vi "beta-3.0.0.vi"() -> ()   [LabVIEW 2016]
uses:
  <vilib>/FPGAPlugInAG/cRIO-9063/niLvFpga_Open_cRIO-9063.vi
  <vilib>/rvi/interface/common/dynamic/niFpgaDynamicAddResources.vi
  <vilib>/Utility/error.llb/Error Cluster From Error Code.vi
  <vilib>/rvi/errors/niLvFpgaAdjustHostInterfaceError.vi
  <vilib>/FPGAPlugInAG/Dynamic/niLvFpga_Close_Dynamic.vi
  <vilib>/rvi/interface/nirviOpenFPGA/nirviOpenFPGA.xnode
  FPGA Bitfiles/multi-functionpr_FPGATarget_multi-function-f_bsn-gyeHrfY.lvbitx
  <vilib>/rvi/interface/nirviReadWriteControl/nirviReadWriteControl.xnode
  <vilib>/rvi/interface/nirviCloseFPGA/nirviCloseFPGA.xnode
  NiFpgaLv.dll
  <vilib>/rvi/interface/Simulation/niFpgaSimulationCallBeginRW.vi
panel:
  out "change indicator":T1
  in  "Output Configuration":T2={"Channel0"={"function"=enum."OFF", "switch high"=3.5, "switch low"=0.0, "scan begin"=0.0, "scan end"=0.0, "scan step"=0.0, "and gate high"=3.5, "and gate low"=0.0, "or gate high"=3.5, "or gate low"=0.0, "main input"=enum."DIO0", "sub input"=enum."DIO0"}, "Channel1"={"function"=enum."OFF", "switch high"=3.5, "switch low"=0.0, "scan begin"=0.0, "scan end"=0.0, "scan step"=0.0, "and gate high"=3.5, "and gate low"=0.0, "or gate high"=3.5, "or gate low"=0.0, "main input"=enum."DIO0", "sub input"=enum."DIO0"}, "Channel2"={"function"=enum."OFF", "switch high"=3.5, "switch low"=0.0, "scan begin"=0.0, "scan end"=0.0, "scan step"=0.0, "and gate high"=3.5, "and gate low"=0.0, "or gate high"=3.5, "or gate low"=0.0, "main input"=enum."DIO0", "sub input"=enum."DIO0"}, "Channel3"={"function"=enum."OFF", "switch high"=3.5, "switch low"=0.0, "scan begin"=0.0, "scan end"=0.0, "scan step"=0.0, "and gate high"=3.5, "and gate low"=0.0, "or gate high"=3.5, "or gate low"=0.0, "main input"=enum."DIO0", "sub input"=enum."DIO0"}, "Channel4"={"function"=enum."OFF", "switch high"=3.5, "switch low"=0.0, "scan begin"=0.0, "scan end"=0.0, "scan step"=0.0, "and gate high"=3.5, "and gate low"=0.0, "or gate high"=3.5, "or gate low"=0.0, "main input"=enum."DIO0", "sub input"=enum."DIO0"}, "Channel5"={"function"=enum."OFF", "switch high"=3.5, "switch low"=0.0, "scan begin"=0.0, "scan end"=0.0, "scan step"=0.0, "and gate high"=3.5, "and gate low"=0.0, "or gate high"=3.5, "or gate low"=0.0, "main input"=enum."DIO0", "sub input"=enum."DIO0"}, "Channel6"={"function"=enum."OFF", "switch high"=3.5, "switch low"=0.0, "scan begin"=0.0, "scan end"=0.0, "scan step"=0.0, "and gate high"=3.5, "and gate low"=0.0, "or gate high"=3.5, "or gate low"=0.0, "main input"=enum."DIO0", "sub input"=enum."DIO0"}, "Channel7"={"function"=enum."OFF", "switch high"=3.5, "switch low"=0.0, "scan begin"=0.0, "scan end"=0.0, "scan step"=0.0, "and gate high"=3.5, "and gate low"=0.0, "or gate high"=3.5, "or gate low"=0.0, "main input"=enum."DIO0", "sub input"=enum."DIO0"}, "Channel8"={"function"=enum."OFF", "switch high"=3.5, "switch low"=0.0, "scan begin"=0.0, "scan end"=0.0, "scan step"=0.0, "and gate high"=3.5, "and gate low"=0.0, "or gate high"=3.5, "or gate low"=0.0, "main input"=enum."DIO0", "sub input"=enum."DIO0"}, "Channel9"={"function"=enum."OFF", "switch high"=3.5, "switch low"=0.0, "scan begin"=0.0, "scan end"=0.0, "scan step"=0.0, "and gate high"=3.5, "and gate low"=0.0, "or gate high"=3.5, "or gate low"=0.0, "main input"=enum."DIO0", "sub input"=enum."DIO0"}, "Channel10"={"function"=enum."OFF", "switch high"=3.5, "switch low"=0.0, "scan begin"=0.0, "scan end"=0.0, "scan step"=0.0, "and gate high"=3.5, "and gate low"=0.0, "or gate high"=3.5, "or gate low"=0.0, "main input"=enum."DIO0", "sub input"=enum."DIO0"}, "Channel11"={"function"=enum."OFF", "switch high"=3.5, "switch low"=0.0, "scan begin"=0.0, "scan end"=0.0, "scan step"=0.0, "and gate high"=3.5, "and gate low"=0.0, "or gate high"=3.5, "or gate low"=0.0, "main input"=enum."DIO0", "sub input"=enum."DIO0"}, "Channel12"={"function"=enum."OFF", "switch high"=3.5, "switch low"=0.0, "scan begin"=0.0, "scan end"=0.0, "scan step"=0.0, "and gate high"=3.5, "and gate low"=0.0, "or gate high"=3.5, "or gate low"=0.0, "main input"=enum."DIO0", "sub input"=enum."DIO0"}, "Channel13"={"function"=enum."OFF", "switch high"=3.5, "switch low"=0.0, "scan begin"=0.0, "scan end"=0.0, "scan step"=0.0, "and gate high"=3.5, "and gate low"=0.0, "or gate high"=3.5, "or gate low"=0.0, "main input"=enum."DIO0", "sub input"=enum."DIO0"}, "Channel14"={"function"=enum."OFF", "switch high"=3.5, "switch low"=0.0, "scan begin"=0.0, "scan end"=0.0, "scan step"=0.0, "and gate high"=3.5, "and gate low"=0.0, "or gate high"=3.5, "or gate low"=0.0, "main input"=enum."DIO0", "sub input"=enum."DIO0"}, "Channel15"={"function"=enum."OFF", "switch high"=3.5, "switch low"=0.0, "scan begin"=0.0, "scan end"=0.0, "scan step"=0.0, "and gate high"=3.5, "and gate low"=0.0, "or gate high"=3.5, "or gate low"=0.0, "main input"=enum."DIO0", "sub input"=enum."DIO0"}} {"Channel15"."or gate low" format="%#_17g"; "Channel15"."or gate high" format="%#_17g"; "Channel15"."and gate low" format="%#_17g"; "Channel15"."and gate high" format="%#_17g"; "Channel15"."scan step" format="%#_17g"; "Channel15"."scan end" format="%#_17g"; "Channel15"."scan begin" format="%#_17g"; "Channel15"."switch low" format="%#_17g"; "Channel15"."switch high" format="%#_17g"; "Channel14"."or gate low" format="%#_17g"; "Channel14"."or gate high" format="%#_17g"; "Channel14"."and gate low" format="%#_17g"; "Channel14"."and gate high" format="%#_17g"; "Channel14"."scan step" format="%#_17g"; "Channel14"."scan end" format="%#_17g"; "Channel14"."scan begin" format="%#_17g"; "Channel14"."switch low" format="%#_17g"; "Channel14"."switch high" format="%#_17g"; "Channel13"."or gate low" format="%#_17g"; "Channel13"."or gate high" format="%#_17g"; "Channel13"."and gate low" format="%#_17g"; "Channel13"."and gate high" format="%#_17g"; "Channel13"."scan step" format="%#_17g"; "Channel13"."scan end" format="%#_17g"; "Channel13"."scan begin" format="%#_17g"; "Channel13"."switch low" format="%#_17g"; "Channel13"."switch high" format="%#_17g"; "Channel12"."or gate low" format="%#_17g"; "Channel12"."or gate high" format="%#_17g"; "Channel12"."and gate low" format="%#_17g"; "Channel12"."and gate high" format="%#_17g"; "Channel12"."scan step" format="%#_17g"; "Channel12"."scan end" format="%#_17g"; "Channel12"."scan begin" format="%#_17g"; "Channel12"."switch low" format="%#_17g"; "Channel12"."switch high" format="%#_17g"; "Channel11"."or gate low" format="%#_17g"; "Channel11"."or gate high" format="%#_17g"; "Channel11"."and gate low" format="%#_17g"; "Channel11"."and gate high" format="%#_17g"; "Channel11"."scan step" format="%#_17g"; "Channel11"."scan end" format="%#_17g"; "Channel11"."scan begin" format="%#_17g"; "Channel11"."switch low" format="%#_17g"; "Channel11"."switch high" format="%#_17g"; "Channel10"."or gate low" format="%#_17g"; "Channel10"."or gate high" format="%#_17g"; "Channel10"."and gate low" format="%#_17g"; "Channel10"."and gate high" format="%#_17g"; "Channel10"."scan step" format="%#_17g"; "Channel10"."scan end" format="%#_17g"; "Channel10"."scan begin" format="%#_17g"; "Channel10"."switch low" format="%#_17g"; "Channel10"."switch high" format="%#_17g"; "Channel9"."or gate low" format="%#_17g"; "Channel9"."or gate high" format="%#_17g"; "Channel9"."and gate low" format="%#_17g"; "Channel9"."and gate high" format="%#_17g"; "Channel9"."scan step" format="%#_17g"; "Channel9"."scan end" format="%#_17g"; "Channel9"."scan begin" format="%#_17g"; "Channel9"."switch low" format="%#_17g"; "Channel9"."switch high" format="%#_17g"; "Channel8"."or gate low" format="%#_17g"; "Channel8"."or gate high" format="%#_17g"; "Channel8"."and gate low" format="%#_17g"; "Channel8"."and gate high" format="%#_17g"; "Channel8"."scan step" format="%#_17g"; "Channel8"."scan end" format="%#_17g"; "Channel8"."scan begin" format="%#_17g"; "Channel8"."switch low" format="%#_17g"; "Channel8"."switch high" format="%#_17g"; "Channel7"."or gate low" format="%#_17g"; "Channel7"."or gate high" format="%#_17g"; "Channel7"."and gate low" format="%#_17g"; "Channel7"."and gate high" format="%#_17g"; "Channel7"."scan step" format="%#_17g"; "Channel7"."scan end" format="%#_17g"; "Channel7"."scan begin" format="%#_17g"; "Channel7"."switch low" format="%#_17g"; "Channel7"."switch high" format="%#_17g"; "Channel6"."or gate low" format="%#_17g"; "Channel6"."or gate high" format="%#_17g"; "Channel6"."and gate low" format="%#_17g"; "Channel6"."and gate high" format="%#_17g"; "Channel6"."scan step" format="%#_17g"; "Channel6"."scan end" format="%#_17g"; "Channel6"."scan begin" format="%#_17g"; "Channel6"."switch low" format="%#_17g"; "Channel6"."switch high" format="%#_17g"; "Channel5"."or gate low" format="%#_17g"; "Channel5"."or gate high" format="%#_17g"; "Channel5"."and gate low" format="%#_17g"; "Channel5"."and gate high" format="%#_17g"; "Channel5"."scan step" format="%#_17g"; "Channel5"."scan end" format="%#_17g"; "Channel5"."scan begin" format="%#_17g"; "Channel5"."switch low" format="%#_17g"; "Channel5"."switch high" format="%#_17g"; "Channel4"."or gate low" format="%#_17g"; "Channel4"."or gate high" format="%#_17g"; "Channel4"."and gate low" format="%#_17g"; "Channel4"."and gate high" format="%#_17g"; "Channel4"."scan step" format="%#_17g"; "Channel4"."scan end" format="%#_17g"; "Channel4"."scan begin" format="%#_17g"; "Channel4"."switch low" format="%#_17g"; "Channel4"."switch high" format="%#_17g"; "Channel3"."or gate low" format="%#_17g"; "Channel3"."or gate high" format="%#_17g"; "Channel3"."and gate low" format="%#_17g"; "Channel3"."and gate high" format="%#_17g"; "Channel3"."scan step" format="%#_17g"; "Channel3"."scan end" format="%#_17g"; "Channel3"."scan begin" format="%#_17g"; "Channel3"."switch low" format="%#_17g"; "Channel3"."switch high" format="%#_17g"; "Channel2"."or gate low" format="%#_17g"; "Channel2"."or gate high" format="%#_17g"; "Channel2"."and gate low" format="%#_17g"; "Channel2"."and gate high" format="%#_17g"; "Channel2"."scan step" format="%#_17g"; "Channel2"."scan end" format="%#_17g"; "Channel2"."scan begin" format="%#_17g"; "Channel2"."switch low" format="%#_17g"; "Channel2"."switch high" format="%#_17g"; "Channel1"."or gate low" format="%#_17g"; "Channel1"."or gate high" format="%#_17g"; "Channel1"."and gate low" format="%#_17g"; "Channel1"."and gate high" format="%#_17g"; "Channel1"."scan step" format="%#_17g"; "Channel1"."scan end" format="%#_17g"; "Channel1"."scan begin" format="%#_17g"; "Channel1"."switch low" format="%#_17g"; "Channel1"."switch high" format="%#_17g"; "Channel0"."or gate low" format="%#_17g"; "Channel0"."or gate high" format="%#_17g"; "Channel0"."and gate low" format="%#_17g"; "Channel0"."and gate high" format="%#_17g"; "Channel0"."scan step" format="%#_17g"; "Channel0"."scan end" format="%#_17g"; "Channel0"."scan begin" format="%#_17g"; "Channel0"."switch low" format="%#_17g"; "Channel0"."switch high" format="%#_17g"}
  in  "Configure":bool
  in  "Load":bool
  out "State":enum16{"Loading", "Running"}(ring)
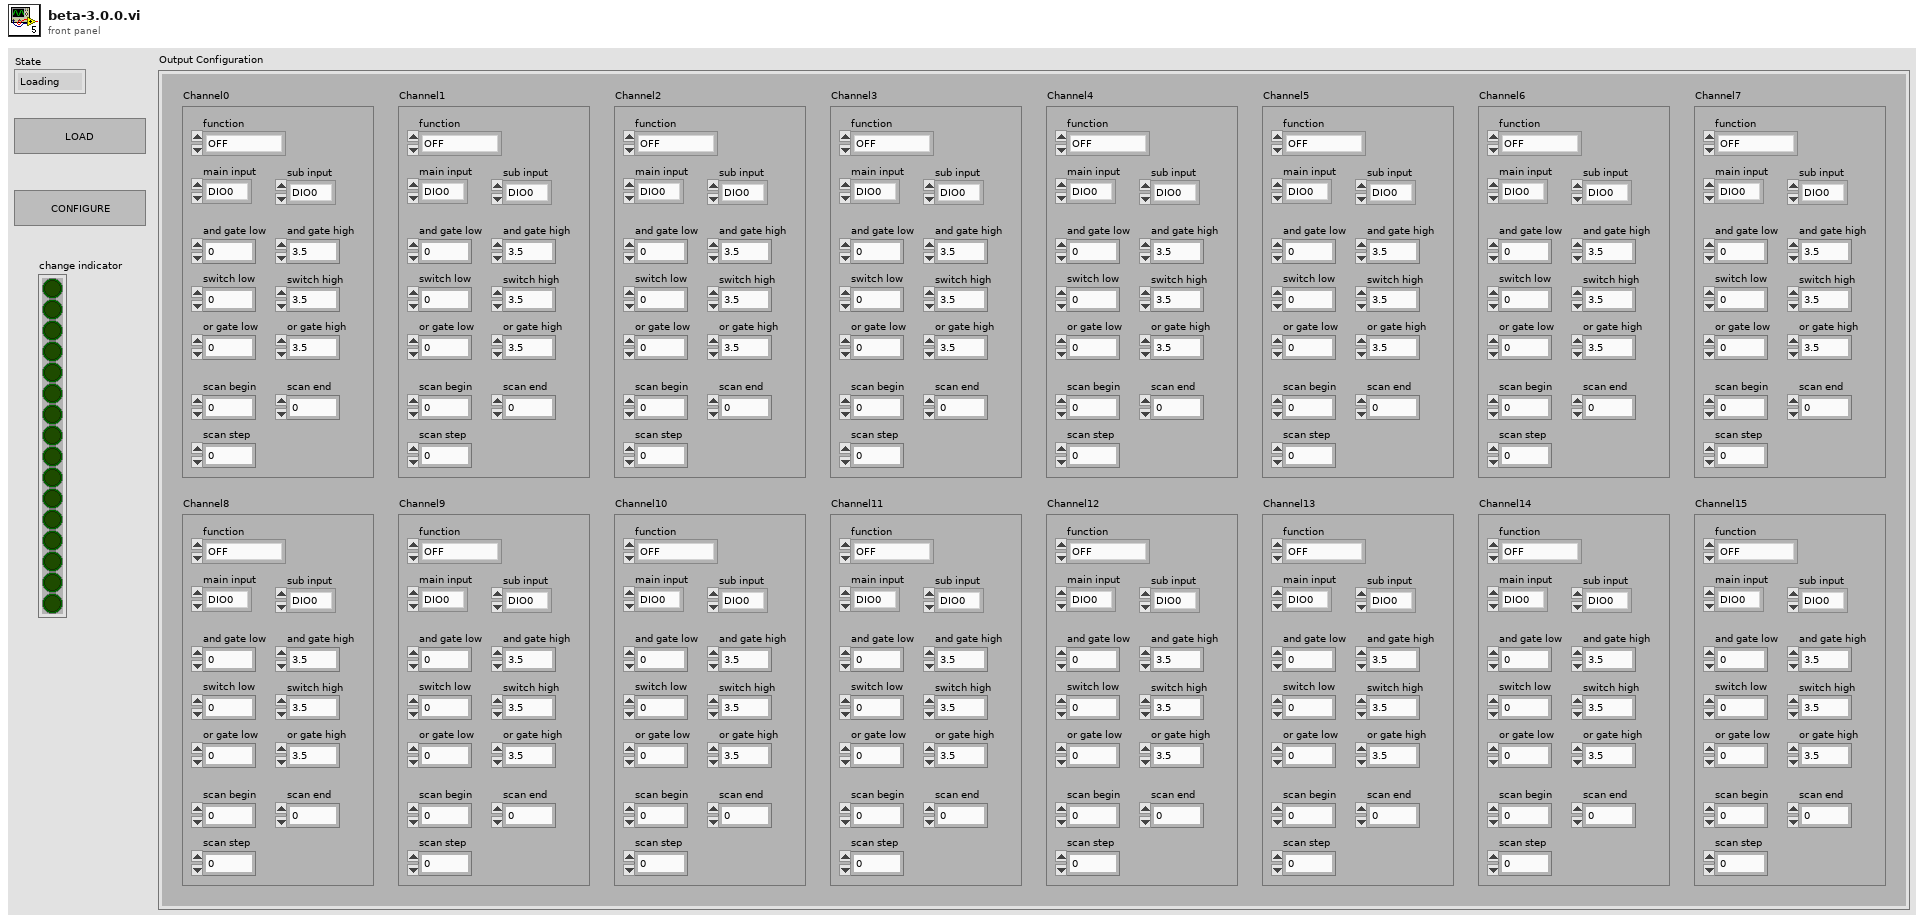
[diagram p1: front panel]
types:
  T1 = cluster{bool, bool, bool, bool, bool, bool, bool, bool, bool, bool, bool, bool, bool, bool, bool, bool}
  T2 = cluster{"Channel0":cluster{"function":enum16{"OFF", "SWITCH", "AND GATE", "OR GATE", "ITERATION"}, "switch high":sgl, "switch low":sgl, "scan begin":sgl, "scan end":sgl, "scan step":sgl, "and gate high":sgl, "and gate low":sgl, "or gate high":sgl, "or gate low":sgl, "main input":enum16{"DIO0", "DIO1", "DIO2", "DIO3", "DIO4", "DIO5", "DIO6", "DIO7", "DIO8", "DIO9", "DIO10", "DIO11", "DIO12", "DIO13", "DIO14", "DIO15", "DIO16", "DIO17", "DIO18", "DIO19", "DIO20", "DIO21", "DIO22", "DIO23", "DIO24", "DIO25", "DIO26", "DIO27", "DIO28", "DIO29", "DIO30", "DIO31"}, "sub input":enum16{"DIO0", "DIO1", "DIO2", "DIO3", "DIO4", "DIO5", "DIO6", "DIO7", "DIO8", "DIO9", "DIO10", "DIO11", "DIO12", "DIO13", "DIO14", "DIO15", "DIO16", "DIO17", "DIO18", "DIO19", "DIO20", "DIO21", "DIO22", "DIO23", "DIO24", "DIO25", "DIO26", "DIO27", "DIO28", "DIO29", "DIO30", "DIO31"}}, "Channel1":cluster{"function":enum16{"OFF", "SWITCH", "AND GATE", "OR GATE", "ITERATION"}, "switch high":sgl, "switch low":sgl, "scan begin":sgl, "scan end":sgl, "scan step":sgl, "and gate high":sgl, "and gate low":sgl, "or gate high":sgl, "or gate low":sgl, "main input":enum16{"DIO0", "DIO1", "DIO2", "DIO3", "DIO4", "DIO5", "DIO6", "DIO7", "DIO8", "DIO9", "DIO10", "DIO11", "DIO12", "DIO13", "DIO14", "DIO15", "DIO16", "DIO17", "DIO18", "DIO19", "DIO20", "DIO21", "DIO22", "DIO23", "DIO24", "DIO25", "DIO26", "DIO27", "DIO28", "DIO29", "DIO30", "DIO31"}, "sub input":enum16{"DIO0", "DIO1", "DIO2", "DIO3", "DIO4", "DIO5", "DIO6", "DIO7", "DIO8", "DIO9", "DIO10", "DIO11", "DIO12", "DIO13", "DIO14", "DIO15", "DIO16", "DIO17", "DIO18", "DIO19", "DIO20", "DIO21", "DIO22", "DIO23", "DIO24", "DIO25", "DIO26", "DIO27", "DIO28", "DIO29", "DIO30", "DIO31"}}, "Channel2":cluster{"function":enum16{"OFF", "SWITCH", "AND GATE", "OR GATE", "ITERATION"}, "switch high":sgl, "switch low":sgl, "scan begin":sgl, "scan end":sgl, "scan step":sgl, "and gate high":sgl, "and gate low":sgl, "or gate high":sgl, "or gate low":sgl, "main input":enum16{"DIO0", "DIO1", "DIO2", "DIO3", "DIO4", "DIO5", "DIO6", "DIO7", "DIO8", "DIO9", "DIO10", "DIO11", "DIO12", "DIO13", "DIO14", "DIO15", "DIO16", "DIO17", "DIO18", "DIO19", "DIO20", "DIO21", "DIO22", "DIO23", "DIO24", "DIO25", "DIO26", "DIO27", "DIO28", "DIO29", "DIO30", "DIO31"}, "sub input":enum16{"DIO0", "DIO1", "DIO2", "DIO3", "DIO4", "DIO5", "DIO6", "DIO7", "DIO8", "DIO9", "DIO10", "DIO11", "DIO12", "DIO13", "DIO14", "DIO15", "DIO16", "DIO17", "DIO18", "DIO19", "DIO20", "DIO21", "DIO22", "DIO23", "DIO24", "DIO25", "DIO26", "DIO27", "DIO28", "DIO29", "DIO30", "DIO31"}}, "Channel3":cluster{"function":enum16{"OFF", "SWITCH", "AND GATE", "OR GATE", "ITERATION"}, "switch high":sgl, "switch low":sgl, "scan begin":sgl, "scan end":sgl, "scan step":sgl, "and gate high":sgl, "and gate low":sgl, "or gate high":sgl, "or gate low":sgl, "main input":enum16{"DIO0", "DIO1", "DIO2", "DIO3", "DIO4", "DIO5", "DIO6", "DIO7", "DIO8", "DIO9", "DIO10", "DIO11", "DIO12", "DIO13", "DIO14", "DIO15", "DIO16", "DIO17", "DIO18", "DIO19", "DIO20", "DIO21", "DIO22", "DIO23", "DIO24", "DIO25", "DIO26", "DIO27", "DIO28", "DIO29", "DIO30", "DIO31"}, "sub input":enum16{"DIO0", "DIO1", "DIO2", "DIO3", "DIO4", "DIO5", "DIO6", "DIO7", "DIO8", "DIO9", "DIO10", "DIO11", "DIO12", "DIO13", "DIO14", "DIO15", "DIO16", "DIO17", "DIO18", "DIO19", "DIO20", "DIO21", "DIO22", "DIO23", "DIO24", "DIO25", "DIO26", "DIO27", "DIO28", "DIO29", "DIO30", "DIO31"}}, "Channel4":cluster{"function":enum16{"OFF", "SWITCH", "AND GATE", "OR GATE", "ITERATION"}, "switch high":sgl, "switch low":sgl, "scan begin":sgl, "scan end":sgl, "scan step":sgl, "and gate high":sgl, "and gate low":sgl, "or gate high":sgl, "or gate low":sgl, "main input":enum16{"DIO0", "DIO1", "DIO2", "DIO3", "DIO4", "DIO5", "DIO6", "DIO7", "DIO8", "DIO9", "DIO10", "DIO11", "DIO12", "DIO13", "DIO14", "DIO15", "DIO16", "DIO17", "DIO18", "DIO19", "DIO20", "DIO21", "DIO22", "DIO23", "DIO24", "DIO25", "DIO26", "DIO27", "DIO28", "DIO29", "DIO30", "DIO31"}, "sub input":enum16{"DIO0", "DIO1", "DIO2", "DIO3", "DIO4", "DIO5", "DIO6", "DIO7", "DIO8", "DIO9", "DIO10", "DIO11", "DIO12", "DIO13", "DIO14", "DIO15", "DIO16", "DIO17", "DIO18", "DIO19", "DIO20", "DIO21", "DIO22", "DIO23", "DIO24", "DIO25", "DIO26", "DIO27", "DIO28", "DIO29", "DIO30", "DIO31"}}, "Channel5":cluster{"function":enum16{"OFF", "SWITCH", "AND GATE", "OR GATE", "ITERATION"}, "switch high":sgl, "switch low":sgl, "scan begin":sgl, "scan end":sgl, "scan step":sgl, "and gate high":sgl, "and gate low":sgl, "or gate high":sgl, "or gate low":sgl, "main input":enum16{"DIO0", "DIO1", "DIO2", "DIO3", "DIO4", "DIO5", "DIO6", "DIO7", "DIO8", "DIO9", "DIO10", "DIO11", "DIO12", "DIO13", "DIO14", "DIO15", "DIO16", "DIO17", "DIO18", "DIO19", "DIO20", "DIO21", "DIO22", "DIO23", "DIO24", "DIO25", "DIO26", "DIO27", "DIO28", "DIO29", "DIO30", "DIO31"}, "sub input":enum16{"DIO0", "DIO1", "DIO2", "DIO3", "DIO4", "DIO5", "DIO6", "DIO7", "DIO8", "DIO9", "DIO10", "DIO11", "DIO12", "DIO13", "DIO14", "DIO15", "DIO16", "DIO17", "DIO18", "DIO19", "DIO20", "DIO21", "DIO22", "DIO23", "DIO24", "DIO25", "DIO26", "DIO27", "DIO28", "DIO29", "DIO30", "DIO31"}}, "Channel6":cluster{"function":enum16{"OFF", "SWITCH", "AND GATE", "OR GATE", "ITERATION"}, "switch high":sgl, "switch low":sgl, "scan begin":sgl, "scan end":sgl, "scan step":sgl, "and gate high":sgl, "and gate low":sgl, "or gate high":sgl, "or gate low":sgl, "main input":enum16{"DIO0", "DIO1", "DIO2", "DIO3", "DIO4", "DIO5", "DIO6", "DIO7", "DIO8", "DIO9", "DIO10", "DIO11", "DIO12", "DIO13", "DIO14", "DIO15", "DIO16", "DIO17", "DIO18", "DIO19", "DIO20", "DIO21", "DIO22", "DIO23", "DIO24", "DIO25", "DIO26", "DIO27", "DIO28", "DIO29", "DIO30", "DIO31"}, "sub input":enum16{"DIO0", "DIO1", "DIO2", "DIO3", "DIO4", "DIO5", "DIO6", "DIO7", "DIO8", "DIO9", "DIO10", "DIO11", "DIO12", "DIO13", "DIO14", "DIO15", "DIO16", "DIO17", "DIO18", "DIO19", "DIO20", "DIO21", "DIO22", "DIO23", "DIO24", "DIO25", "DIO26", "DIO27", "DIO28", "DIO29", "DIO30", "DIO31"}}, "Channel7":cluster{"function":enum16{"OFF", "SWITCH", "AND GATE", "OR GATE", "ITERATION"}, "switch high":sgl, "switch low":sgl, "scan begin":sgl, "scan end":sgl, "scan step":sgl, "and gate high":sgl, "and gate low":sgl, "or gate high":sgl, "or gate low":sgl, "main input":enum16{"DIO0", "DIO1", "DIO2", "DIO3", "DIO4", "DIO5", "DIO6", "DIO7", "DIO8", "DIO9", "DIO10", "DIO11", "DIO12", "DIO13", "DIO14", "DIO15", "DIO16", "DIO17", "DIO18", "DIO19", "DIO20", "DIO21", "DIO22", "DIO23", "DIO24", "DIO25", "DIO26", "DIO27", "DIO28", "DIO29", "DIO30", "DIO31"}, "sub input":enum16{"DIO0", "DIO1", "DIO2", "DIO3", "DIO4", "DIO5", "DIO6", "DIO7", "DIO8", "DIO9", "DIO10", "DIO11", "DIO12", "DIO13", "DIO14", "DIO15", "DIO16", "DIO17", "DIO18", "DIO19", "DIO20", "DIO21", "DIO22", "DIO23", "DIO24", "DIO25", "DIO26", "DIO27", "DIO28", "DIO29", "DIO30", "DIO31"}}, "Channel8":cluster{"function":enum16{"OFF", "SWITCH", "AND GATE", "OR GATE", "ITERATION"}, "switch high":sgl, "switch low":sgl, "scan begin":sgl, "scan end":sgl, "scan step":sgl, "and gate high":sgl, "and gate low":sgl, "or gate high":sgl, "or gate low":sgl, "main input":enum16{"DIO0", "DIO1", "DIO2", "DIO3", "DIO4", "DIO5", "DIO6", "DIO7", "DIO8", "DIO9", "DIO10", "DIO11", "DIO12", "DIO13", "DIO14", "DIO15", "DIO16", "DIO17", "DIO18", "DIO19", "DIO20", "DIO21", "DIO22", "DIO23", "DIO24", "DIO25", "DIO26", "DIO27", "DIO28", "DIO29", "DIO30", "DIO31"}, "sub input":enum16{"DIO0", "DIO1", "DIO2", "DIO3", "DIO4", "DIO5", "DIO6", "DIO7", "DIO8", "DIO9", "DIO10", "DIO11", "DIO12", "DIO13", "DIO14", "DIO15", "DIO16", "DIO17", "DIO18", "DIO19", "DIO20", "DIO21", "DIO22", "DIO23", "DIO24", "DIO25", "DIO26", "DIO27", "DIO28", "DIO29", "DIO30", "DIO31"}}, "Channel9":cluster{"function":enum16{"OFF", "SWITCH", "AND GATE", "OR GATE", "ITERATION"}, "switch high":sgl, "switch low":sgl, "scan begin":sgl, "scan end":sgl, "scan step":sgl, "and gate high":sgl, "and gate low":sgl, "or gate high":sgl, "or gate low":sgl, "main input":enum16{"DIO0", "DIO1", "DIO2", "DIO3", "DIO4", "DIO5", "DIO6", "DIO7", "DIO8", "DIO9", "DIO10", "DIO11", "DIO12", "DIO13", "DIO14", "DIO15", "DIO16", "DIO17", "DIO18", "DIO19", "DIO20", "DIO21", "DIO22", "DIO23", "DIO24", "DIO25", "DIO26", "DIO27", "DIO28", "DIO29", "DIO30", "DIO31"}, "sub input":enum16{"DIO0", "DIO1", "DIO2", "DIO3", "DIO4", "DIO5", "DIO6", "DIO7", "DIO8", "DIO9", "DIO10", "DIO11", "DIO12", "DIO13", "DIO14", "DIO15", "DIO16", "DIO17", "DIO18", "DIO19", "DIO20", "DIO21", "DIO22", "DIO23", "DIO24", "DIO25", "DIO26", "DIO27", "DIO28", "DIO29", "DIO30", "DIO31"}}, "Channel10":cluster{"function":enum16{"OFF", "SWITCH", "AND GATE", "OR GATE", "ITERATION"}, "switch high":sgl, "switch low":sgl, "scan begin":sgl, "scan end":sgl, "scan step":sgl, "and gate high":sgl, "and gate low":sgl, "or gate high":sgl, "or gate low":sgl, "main input":enum16{"DIO0", "DIO1", "DIO2", "DIO3", "DIO4", "DIO5", "DIO6", "DIO7", "DIO8", "DIO9", "DIO10", "DIO11", "DIO12", "DIO13", "DIO14", "DIO15", "DIO16", "DIO17", "DIO18", "DIO19", "DIO20", "DIO21", "DIO22", "DIO23", "DIO24", "DIO25", "DIO26", "DIO27", "DIO28", "DIO29", "DIO30", "DIO31"}, "sub input":enum16{"DIO0", "DIO1", "DIO2", "DIO3", "DIO4", "DIO5", "DIO6", "DIO7", "DIO8", "DIO9", "DIO10", "DIO11", "DIO12", "DIO13", "DIO14", "DIO15", "DIO16", "DIO17", "DIO18", "DIO19", "DIO20", "DIO21", "DIO22", "DIO23", "DIO24", "DIO25", "DIO26", "DIO27", "DIO28", "DIO29", "DIO30", "DIO31"}}, "Channel11":cluster{"function":enum16{"OFF", "SWITCH", "AND GATE", "OR GATE", "ITERATION"}, "switch high":sgl, "switch low":sgl, "scan begin":sgl, "scan end":sgl, "scan step":sgl, "and gate high":sgl, "and gate low":sgl, "or gate high":sgl, "or gate low":sgl, "main input":enum16{"DIO0", "DIO1", "DIO2", "DIO3", "DIO4", "DIO5", "DIO6", "DIO7", "DIO8", "DIO9", "DIO10", "DIO11", "DIO12", "DIO13", "DIO14", "DIO15", "DIO16", "DIO17", "DIO18", "DIO19", "DIO20", "DIO21", "DIO22", "DIO23", "DIO24", "DIO25", "DIO26", "DIO27", "DIO28", "DIO29", "DIO30", "DIO31"}, "sub input":enum16{"DIO0", "DIO1", "DIO2", "DIO3", "DIO4", "DIO5", "DIO6", "DIO7", "DIO8", "DIO9", "DIO10", "DIO11", "DIO12", "DIO13", "DIO14", "DIO15", "DIO16", "DIO17", "DIO18", "DIO19", "DIO20", "DIO21", "DIO22", "DIO23", "DIO24", "DIO25", "DIO26", "DIO27", "DIO28", "DIO29", "DIO30", "DIO31"}}, "Channel12":cluster{"function":enum16{"OFF", "SWITCH", "AND GATE", "OR GATE", "ITERATION"}, "switch high":sgl, "switch low":sgl, "scan begin":sgl, "scan end":sgl, "scan step":sgl, "and gate high":sgl, "and gate low":sgl, "or gate high":sgl, "or gate low":sgl, "main input":enum16{"DIO0", "DIO1", "DIO2", "DIO3", "DIO4", "DIO5", "DIO6", "DIO7", "DIO8", "DIO9", "DIO10", "DIO11", "DIO12", "DIO13", "DIO14", "DIO15", "DIO16", "DIO17", "DIO18", "DIO19", "DIO20", "DIO21", "DIO22", "DIO23", "DIO24", "DIO25", "DIO26", "DIO27", "DIO28", "DIO29", "DIO30", "DIO31"}, "sub input":enum16{"DIO0", "DIO1", "DIO2", "DIO3", "DIO4", "DIO5", "DIO6", "DIO7", "DIO8", "DIO9", "DIO10", "DIO11", "DIO12", "DIO13", "DIO14", "DIO15", "DIO16", "DIO17", "DIO18", "DIO19", "DIO20", "DIO21", "DIO22", "DIO23", "DIO24", "DIO25", "DIO26", "DIO27", "DIO28", "DIO29", "DIO30", "DIO31"}}, "Channel13":cluster{"function":enum16{"OFF", "SWITCH", "AND GATE", "OR GATE", "ITERATION"}, "switch high":sgl, "switch low":sgl, "scan begin":sgl, "scan end":sgl, "scan step":sgl, "and gate high":sgl, "and gate low":sgl, "or gate high":sgl, "or gate low":sgl, "main input":enum16{"DIO0", "DIO1", "DIO2", "DIO3", "DIO4", "DIO5", "DIO6", "DIO7", "DIO8", "DIO9", "DIO10", "DIO11", "DIO12", "DIO13", "DIO14", "DIO15", "DIO16", "DIO17", "DIO18", "DIO19", "DIO20", "DIO21", "DIO22", "DIO23", "DIO24", "DIO25", "DIO26", "DIO27", "DIO28", "DIO29", "DIO30", "DIO31"}, "sub input":enum16{"DIO0", "DIO1", "DIO2", "DIO3", "DIO4", "DIO5", "DIO6", "DIO7", "DIO8", "DIO9", "DIO10", "DIO11", "DIO12", "DIO13", "DIO14", "DIO15", "DIO16", "DIO17", "DIO18", "DIO19", "DIO20", "DIO21", "DIO22", "DIO23", "DIO24", "DIO25", "DIO26", "DIO27", "DIO28", "DIO29", "DIO30", "DIO31"}}, "Channel14":cluster{"function":enum16{"OFF", "SWITCH", "AND GATE", "OR GATE", "ITERATION"}, "switch high":sgl, "switch low":sgl, "scan begin":sgl, "scan end":sgl, "scan step":sgl, "and gate high":sgl, "and gate low":sgl, "or gate high":sgl, "or gate low":sgl, "main input":enum16{"DIO0", "DIO1", "DIO2", "DIO3", "DIO4", "DIO5", "DIO6", "DIO7", "DIO8", "DIO9", "DIO10", "DIO11", "DIO12", "DIO13", "DIO14", "DIO15", "DIO16", "DIO17", "DIO18", "DIO19", "DIO20", "DIO21", "DIO22", "DIO23", "DIO24", "DIO25", "DIO26", "DIO27", "DIO28", "DIO29", "DIO30", "DIO31"}, "sub input":enum16{"DIO0", "DIO1", "DIO2", "DIO3", "DIO4", "DIO5", "DIO6", "DIO7", "DIO8", "DIO9", "DIO10", "DIO11", "DIO12", "DIO13", "DIO14", "DIO15", "DIO16", "DIO17", "DIO18", "DIO19", "DIO20", "DIO21", "DIO22", "DIO23", "DIO24", "DIO25", "DIO26", "DIO27", "DIO28", "DIO29", "DIO30", "DIO31"}}, "Channel15":cluster{"function":enum16{"OFF", "SWITCH", "AND GATE", "OR GATE", "ITERATION"}, "switch high":sgl, "switch low":sgl, "scan begin":sgl, "scan end":sgl, "scan step":sgl, "and gate high":sgl, "and gate low":sgl, "or gate high":sgl, "or gate low":sgl, "main input":enum16{"DIO0", "DIO1", "DIO2", "DIO3", "DIO4", "DIO5", "DIO6", "DIO7", "DIO8", "DIO9", "DIO10", "DIO11", "DIO12", "DIO13", "DIO14", "DIO15", "DIO16", "DIO17", "DIO18", "DIO19", "DIO20", "DIO21", "DIO22", "DIO23", "DIO24", "DIO25", "DIO26", "DIO27", "DIO28", "DIO29", "DIO30", "DIO31"}, "sub input":enum16{"DIO0", "DIO1", "DIO2", "DIO3", "DIO4", "DIO5", "DIO6", "DIO7", "DIO8", "DIO9", "DIO10", "DIO11", "DIO12", "DIO13", "DIO14", "DIO15", "DIO16", "DIO17", "DIO18", "DIO19", "DIO20", "DIO21", "DIO22", "DIO23", "DIO24", "DIO25", "DIO26", "DIO27", "DIO28", "DIO29", "DIO30", "DIO31"}}}
  T3 = cluster{"Channel0":cluster{"function":bool, "switch high":bool, "switch low":bool, "scan begin":bool, "scan end":bool, "scan step":bool, "and gate high":bool, "and gate low":bool, "or gate high":bool, "or gate low":bool, "main input":bool, "sub input":bool}, "Channel1":cluster{"function":bool, "switch high":bool, "switch low":bool, "scan begin":bool, "scan end":bool, "scan step":bool, "and gate high":bool, "and gate low":bool, "or gate high":bool, "or gate low":bool, "main input":bool, "sub input":bool}, "Channel2":cluster{"function":bool, "switch high":bool, "switch low":bool, "scan begin":bool, "scan end":bool, "scan step":bool, "and gate high":bool, "and gate low":bool, "or gate high":bool, "or gate low":bool, "main input":bool, "sub input":bool}, "Channel3":cluster{"function":bool, "switch high":bool, "switch low":bool, "scan begin":bool, "scan end":bool, "scan step":bool, "and gate high":bool, "and gate low":bool, "or gate high":bool, "or gate low":bool, "main input":bool, "sub input":bool}, "Channel4":cluster{"function":bool, "switch high":bool, "switch low":bool, "scan begin":bool, "scan end":bool, "scan step":bool, "and gate high":bool, "and gate low":bool, "or gate high":bool, "or gate low":bool, "main input":bool, "sub input":bool}, "Channel5":cluster{"function":bool, "switch high":bool, "switch low":bool, "scan begin":bool, "scan end":bool, "scan step":bool, "and gate high":bool, "and gate low":bool, "or gate high":bool, "or gate low":bool, "main input":bool, "sub input":bool}, "Channel6":cluster{"function":bool, "switch high":bool, "switch low":bool, "scan begin":bool, "scan end":bool, "scan step":bool, "and gate high":bool, "and gate low":bool, "or gate high":bool, "or gate low":bool, "main input":bool, "sub input":bool}, "Channel7":cluster{"function":bool, "switch high":bool, "switch low":bool, "scan begin":bool, "scan end":bool, "scan step":bool, "and gate high":bool, "and gate low":bool, "or gate high":bool, "or gate low":bool, "main input":bool, "sub input":bool}, "Channel8":cluster{"function":bool, "switch high":bool, "switch low":bool, "scan begin":bool, "scan end":bool, "scan step":bool, "and gate high":bool, "and gate low":bool, "or gate high":bool, "or gate low":bool, "main input":bool, "sub input":bool}, "Channel9":cluster{"function":bool, "switch high":bool, "switch low":bool, "scan begin":bool, "scan end":bool, "scan step":bool, "and gate high":bool, "and gate low":bool, "or gate high":bool, "or gate low":bool, "main input":bool, "sub input":bool}, "Channel10":cluster{"function":bool, "switch high":bool, "switch low":bool, "scan begin":bool, "scan end":bool, "scan step":bool, "and gate high":bool, "and gate low":bool, "or gate high":bool, "or gate low":bool, "main input":bool, "sub input":bool}, "Channel11":cluster{"function":bool, "switch high":bool, "switch low":bool, "scan begin":bool, "scan end":bool, "scan step":bool, "and gate high":bool, "and gate low":bool, "or gate high":bool, "or gate low":bool, "main input":bool, "sub input":bool}, "Channel12":cluster{"function":bool, "switch high":bool, "switch low":bool, "scan begin":bool, "scan end":bool, "scan step":bool, "and gate high":bool, "and gate low":bool, "or gate high":bool, "or gate low":bool, "main input":bool, "sub input":bool}, "Channel13":cluster{"function":bool, "switch high":bool, "switch low":bool, "scan begin":bool, "scan end":bool, "scan step":bool, "and gate high":bool, "and gate low":bool, "or gate high":bool, "or gate low":bool, "main input":bool, "sub input":bool}, "Channel14":cluster{"function":bool, "switch high":bool, "switch low":bool, "scan begin":bool, "scan end":bool, "scan step":bool, "and gate high":bool, "and gate low":bool, "or gate high":bool, "or gate low":bool, "main input":bool, "sub input":bool}, "Channel15":cluster{"function":bool, "switch high":bool, "switch low":bool, "scan begin":bool, "scan end":bool, "scan step":bool, "and gate high":bool, "and gate low":bool, "or gate high":bool, "or gate low":bool, "main input":bool, "sub input":bool}}
  T4 = cluster{"function":bool, "switch high":bool, "switch low":bool, "scan begin":bool, "scan end":bool, "scan step":bool, "and gate high":bool, "and gate low":bool, "or gate high":bool, "or gate low":bool, "main input":bool, "sub input":bool}
  T5 = cluster{"function":enum16{"OFF", "SWITCH", "AND GATE", "OR GATE", "ITERATION"}, "switch high":sgl, "switch low":sgl, "scan begin":sgl, "scan end":sgl, "scan step":sgl, "and gate high":sgl, "and gate low":sgl, "or gate high":sgl, "or gate low":sgl, "main input":enum16{"DIO0", "DIO1", "DIO2", "DIO3", "DIO4", "DIO5", "DIO6", "DIO7", "DIO8", "DIO9", "DIO10", "DIO11", "DIO12", "DIO13", "DIO14", "DIO15", "DIO16", "DIO17", "DIO18", "DIO19", "DIO20", "DIO21", "DIO22", "DIO23", "DIO24", "DIO25", "DIO26", "DIO27", "DIO28", "DIO29", "DIO30", "DIO31"}, "sub input":enum16{"DIO0", "DIO1", "DIO2", "DIO3", "DIO4", "DIO5", "DIO6", "DIO7", "DIO8", "DIO9", "DIO10", "DIO11", "DIO12", "DIO13", "DIO14", "DIO15", "DIO16", "DIO17", "DIO18", "DIO19", "DIO20", "DIO21", "DIO22", "DIO23", "DIO24", "DIO25", "DIO26", "DIO27", "DIO28", "DIO29", "DIO30", "DIO31"}}
  T6 = enum16{"OFF", "SWITCH", "AND GATE", "OR GATE", "ITERATION"}
  T7 = enum16{"DIO0", "DIO1", "DIO2", "DIO3", "DIO4", "DIO5", "DIO6", "DIO7", "DIO8", "DIO9", "DIO10", "DIO11", "DIO12", "DIO13", "DIO14", "DIO15", "DIO16", "DIO17", "DIO18", "DIO19", "DIO20", "DIO21", "DIO22", "DIO23", "DIO24", "DIO25", "DIO26", "DIO27", "DIO28", "DIO29", "DIO30", "DIO31"}
  T8 = cluster{"function":enum16{"OFF", "SWITCH", "AND GATE", "OR GATE", "ITERATION"}, "scan end":sgl, "scan begin":sgl, "scan step":sgl, bool, "main input":enum16{"DIO0", "DIO1", "DIO2", "DIO3", "DIO4", "DIO5", "DIO6", "DIO7", "DIO8", "DIO9", "DIO10", "DIO11", "DIO12", "DIO13", "DIO14", "DIO15", "DIO16", "DIO17", "DIO18", "DIO19", "DIO20", "DIO21", "DIO22", "DIO23", "DIO24", "DIO25", "DIO26", "DIO27", "DIO28", "DIO29", "DIO30", "DIO31"}, "sub input":enum16{"DIO0", "DIO1", "DIO2", "DIO3", "DIO4", "DIO5", "DIO6", "DIO7", "DIO8", "DIO9", "DIO10", "DIO11", "DIO12", "DIO13", "DIO14", "DIO15", "DIO16", "DIO17", "DIO18", "DIO19", "DIO20", "DIO21", "DIO22", "DIO23", "DIO24", "DIO25", "DIO26", "DIO27", "DIO28", "DIO29", "DIO30", "DIO31"}}
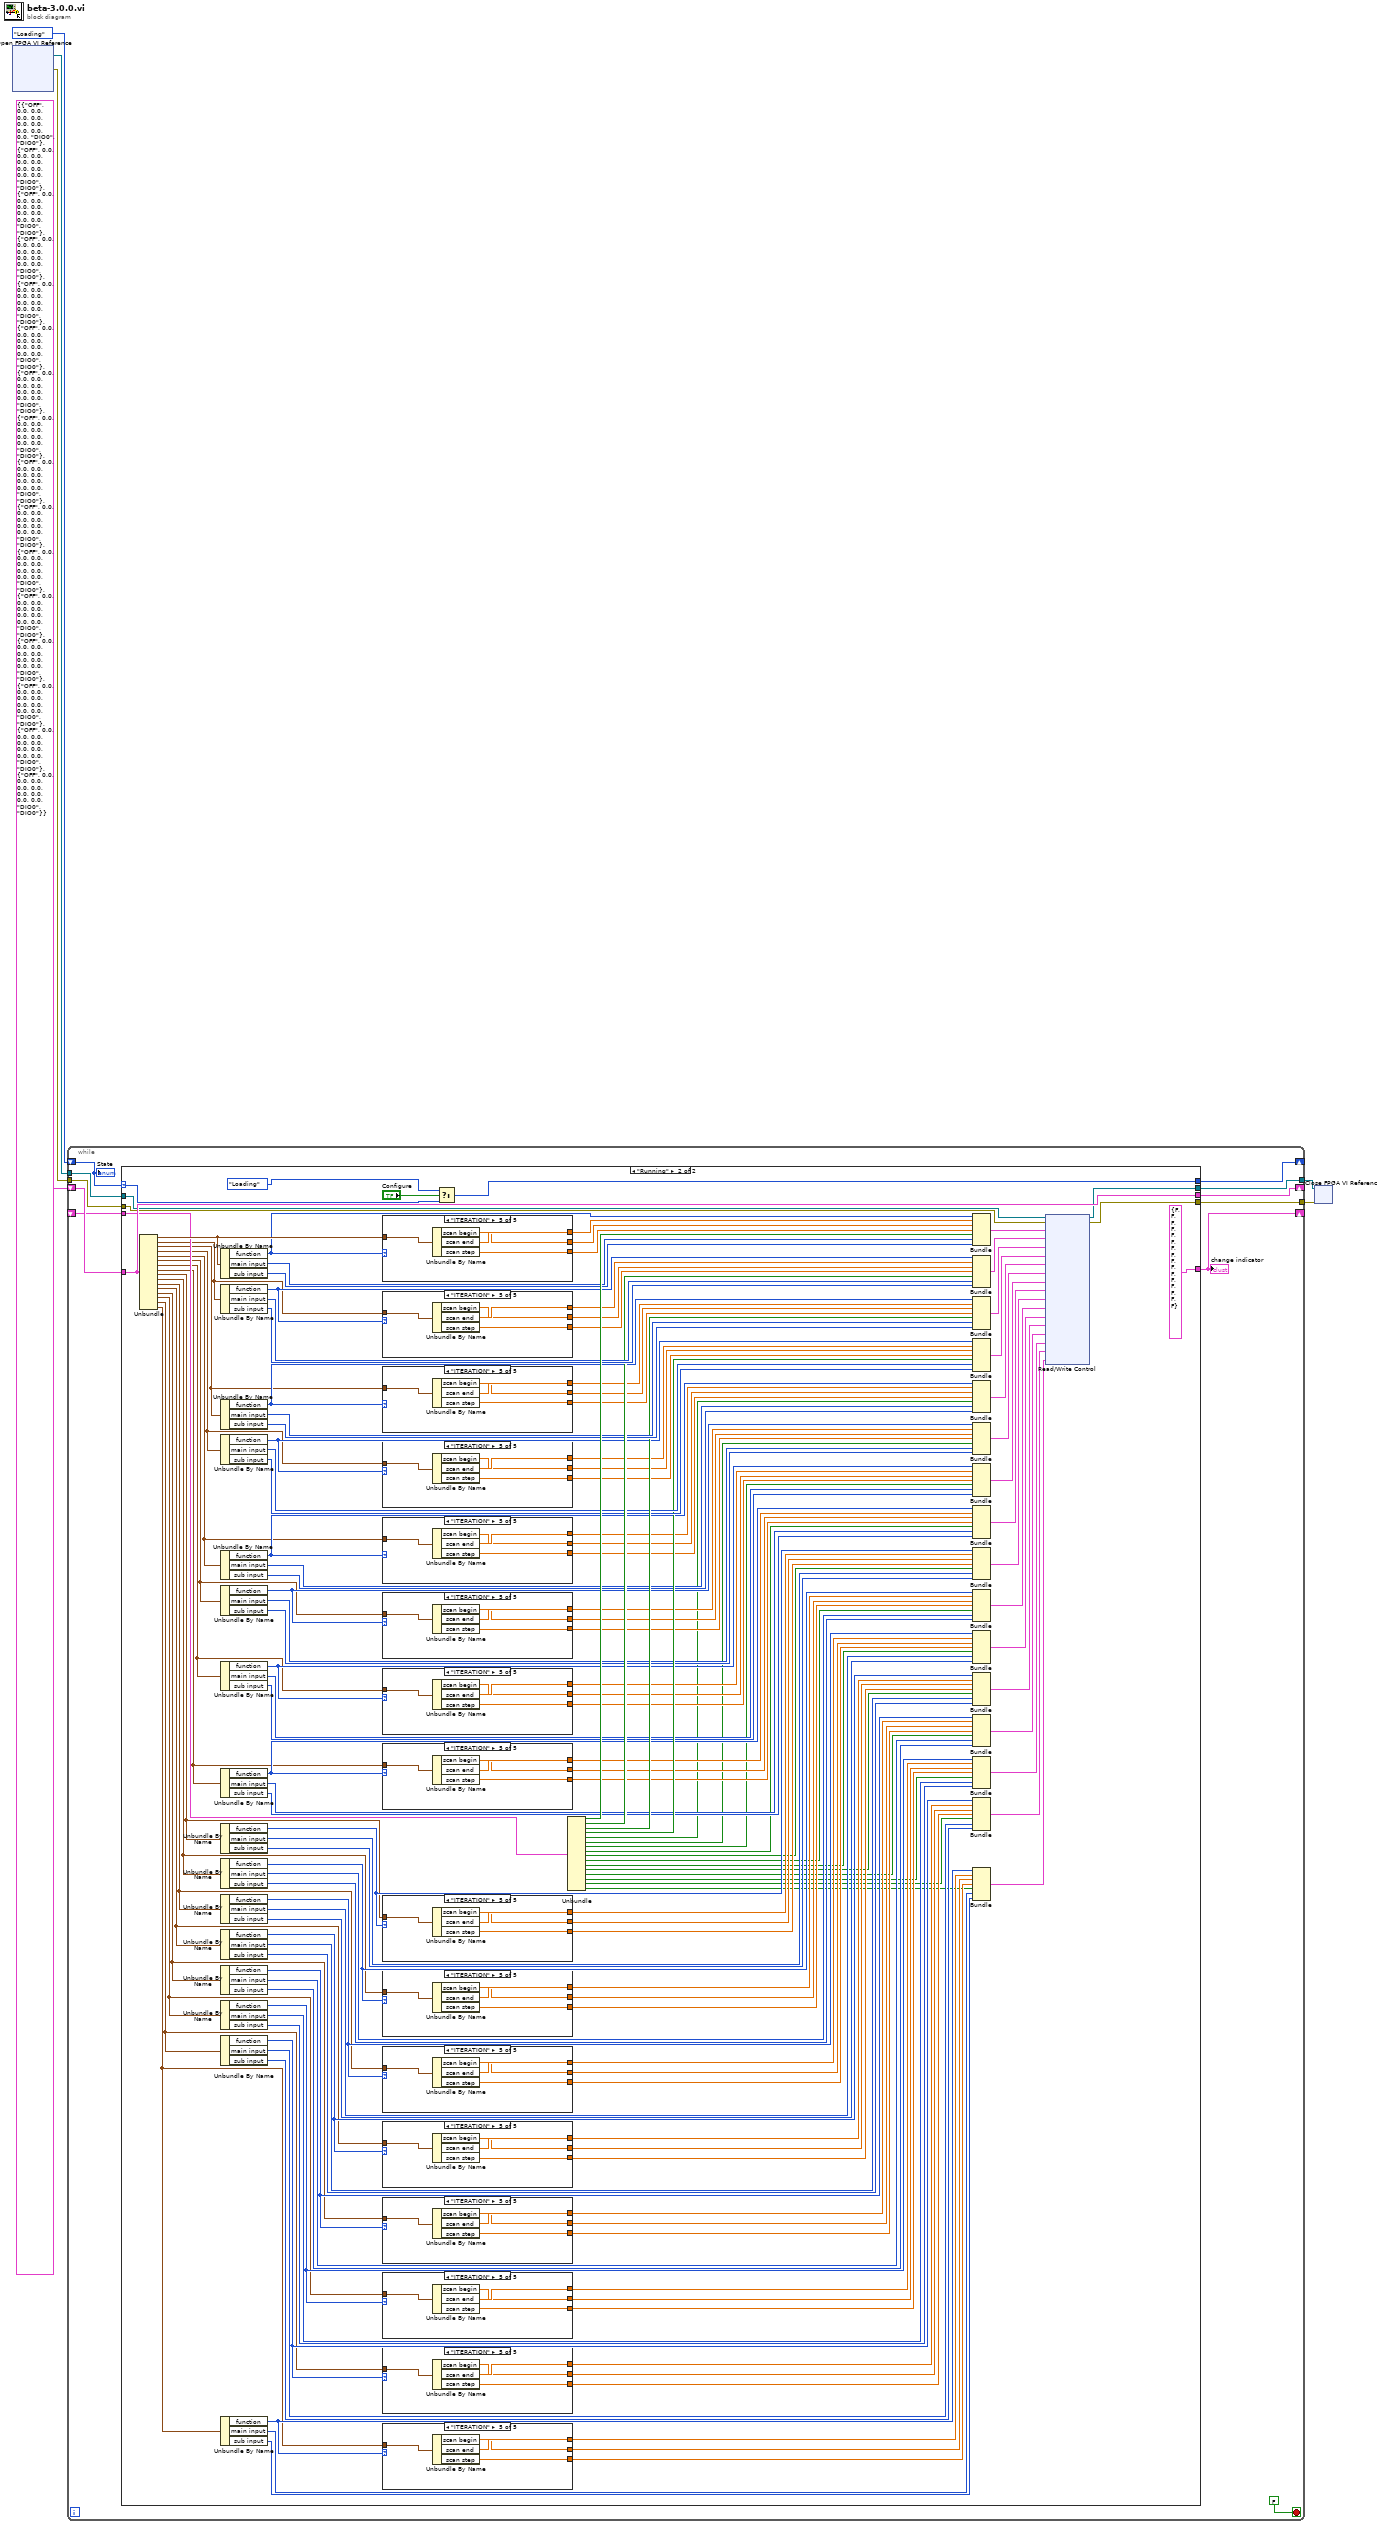
[diagram p0: block diagram]
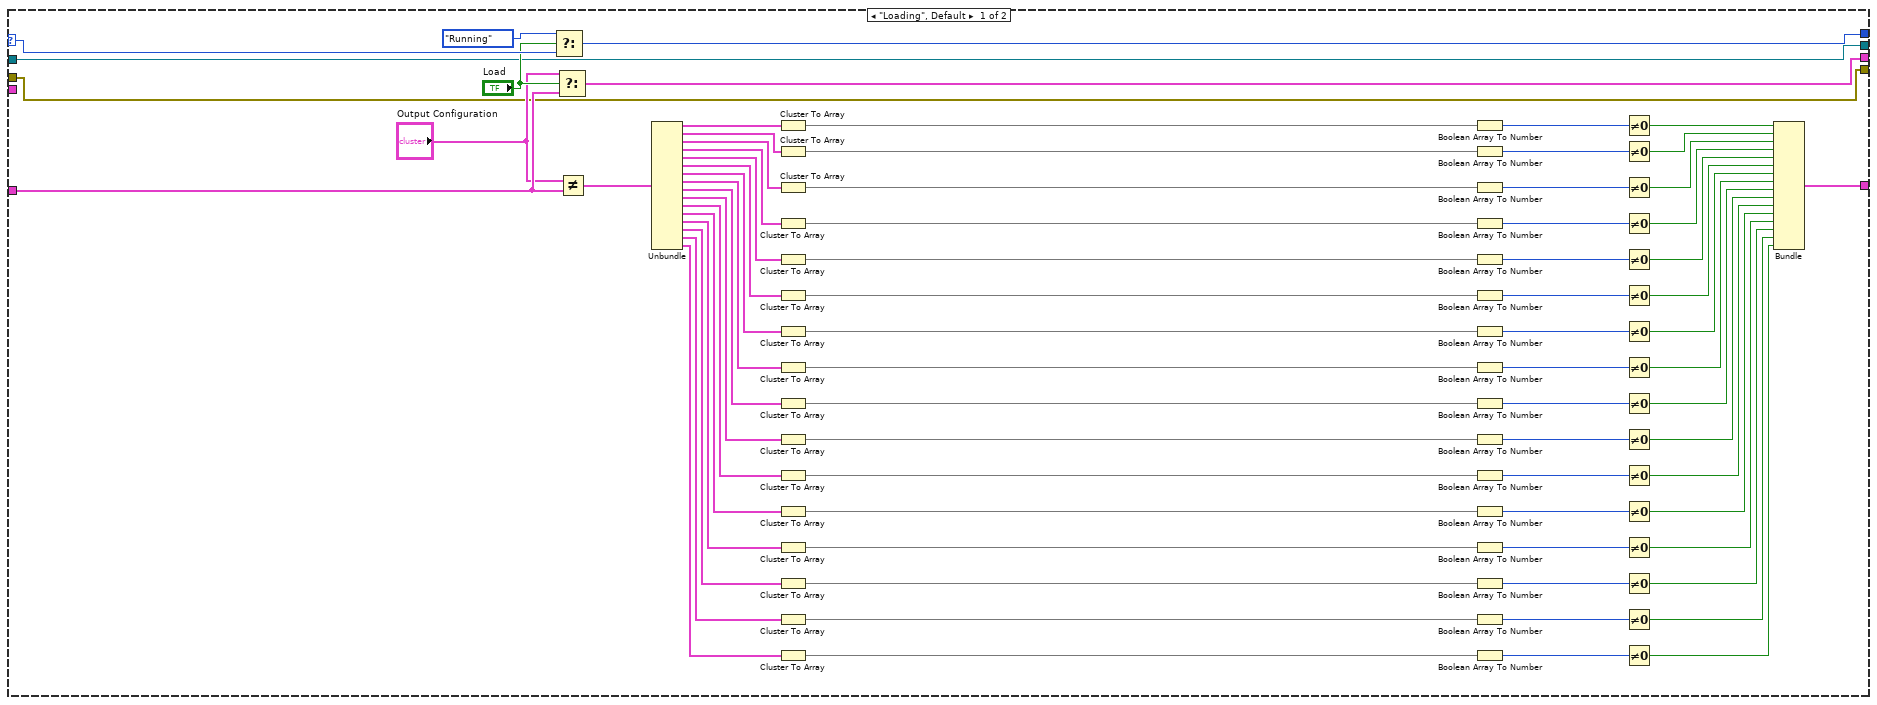
[diagram p2: hidden frame]
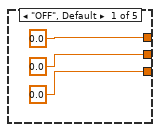
[diagram p3: hidden frame]
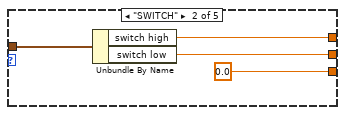
[diagram p4: hidden frame]
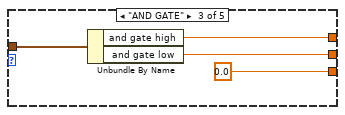
[diagram p5: hidden frame]
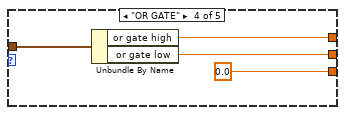
[diagram p6: hidden frame]
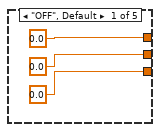
[diagram p7: hidden frame]
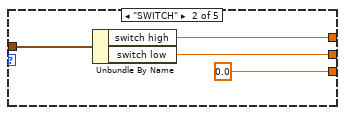
[diagram p8: hidden frame]
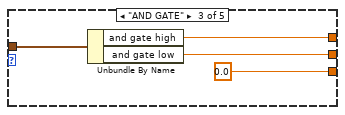
[diagram p9: hidden frame]
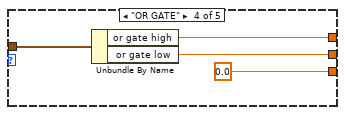
[diagram p10: hidden frame]
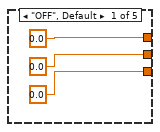
[diagram p11: hidden frame]
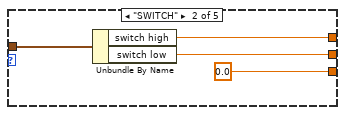
[diagram p12: hidden frame]
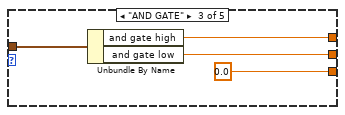
[diagram p13: hidden frame]
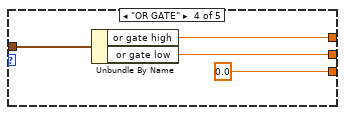
[diagram p14: hidden frame]
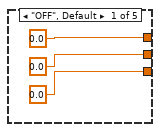
[diagram p15: hidden frame]
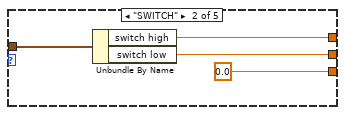
[diagram p16: hidden frame]
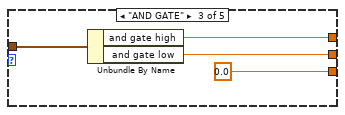
[diagram p17: hidden frame]
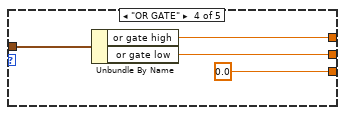
[diagram p18: hidden frame]
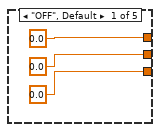
[diagram p19: hidden frame]
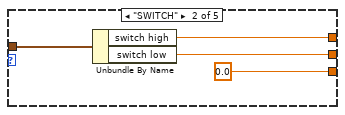
[diagram p20: hidden frame]
diagram:
  n1 = xnode "Open FPGA VI Reference"() -> ("FPGA VI Reference Out"=w4:refnum<k20>, "error out"=w3:errorcluster)  [unwired: 2 in]
  n2 = while {
    shift-right: [w14] -> _
    shift-left: T2 {"Channel0"={"function"=enum."OFF", "switch high"=0.0, "switch low"=0.0, "scan begin"=0.0, "scan end"=0.0, "scan step"=0.0, "and gate high"=0.0, "and gate low"=0.0, "or gate high"=0.0, "or gate low"=0.0, "main input"=enum."DIO0", "sub input"=enum."DIO0"}, "Channel1"={"function"=enum."OFF", "switch high"=0.0, "switch low"=0.0, "scan begin"=0.0, "scan end"=0.0, "scan step"=0.0, "and gate high"=0.0, "and gate low"=0.0, "or gate high"=0.0, "or gate low"=0.0, "main input"=enum."DIO0", "sub input"=enum."DIO0"}, "Channel2"={"function"=enum."OFF", "switch high"=0.0, "switch low"=0.0, "scan begin"=0.0, "scan end"=0.0, "scan step"=0.0, "and gate high"=0.0, "and gate low"=0.0, "or gate high"=0.0, "or gate low"=0.0, "main input"=enum."DIO0", "sub input"=enum."DIO0"}, "Channel3"={"function"=enum."OFF", "switch high"=0.0, "switch low"=0.0, "scan begin"=0.0, "scan end"=0.0, "scan step"=0.0, "and gate high"=0.0, "and gate low"=0.0, "or gate high"=0.0, "or gate low"=0.0, "main input"=enum."DIO0", "sub input"=enum."DIO0"}, "Channel4"={"function"=enum."OFF", "switch high"=0.0, "switch low"=0.0, "scan begin"=0.0, "scan end"=0.0, "scan step"=0.0, "and gate high"=0.0, "and gate low"=0.0, "or gate high"=0.0, "or gate low"=0.0, "main input"=enum."DIO0", "sub input"=enum."DIO0"}, "Channel5"={"function"=enum."OFF", "switch high"=0.0, "switch low"=0.0, "scan begin"=0.0, "scan end"=0.0, "scan step"=0.0, "and gate high"=0.0, "and gate low"=0.0, "or gate high"=0.0, "or gate low"=0.0, "main input"=enum."DIO0", "sub input"=enum."DIO0"}, "Channel6"={"function"=enum."OFF", "switch high"=0.0, "switch low"=0.0, "scan begin"=0.0, "scan end"=0.0, "scan step"=0.0, "and gate high"=0.0, "and gate low"=0.0, "or gate high"=0.0, "or gate low"=0.0, "main input"=enum."DIO0", "sub input"=enum."DIO0"}, "Channel7"={"function"=enum."OFF", "switch high"=0.0, "switch low"=0.0, "scan begin"=0.0, "scan end"=0.0, "scan step"=0.0, "and gate high"=0.0, "and gate low"=0.0, "or gate high"=0.0, "or gate low"=0.0, "main input"=enum."DIO0", "sub input"=enum."DIO0"}, "Channel8"={"function"=enum."OFF", "switch high"=0.0, "switch low"=0.0, "scan begin"=0.0, "scan end"=0.0, "scan step"=0.0, "and gate high"=0.0, "and gate low"=0.0, "or gate high"=0.0, "or gate low"=0.0, "main input"=enum."DIO0", "sub input"=enum."DIO0"}, "Channel9"={"function"=enum."OFF", "switch high"=0.0, "switch low"=0.0, "scan begin"=0.0, "scan end"=0.0, "scan step"=0.0, "and gate high"=0.0, "and gate low"=0.0, "or gate high"=0.0, "or gate low"=0.0, "main input"=enum."DIO0", "sub input"=enum."DIO0"}, "Channel10"={"function"=enum."OFF", "switch high"=0.0, "switch low"=0.0, "scan begin"=0.0, "scan end"=0.0, "scan step"=0.0, "and gate high"=0.0, "and gate low"=0.0, "or gate high"=0.0, "or gate low"=0.0, "main input"=enum."DIO0", "sub input"=enum."DIO0"}, "Channel11"={"function"=enum."OFF", "switch high"=0.0, "switch low"=0.0, "scan begin"=0.0, "scan end"=0.0, "scan step"=0.0, "and gate high"=0.0, "and gate low"=0.0, "or gate high"=0.0, "or gate low"=0.0, "main input"=enum."DIO0", "sub input"=enum."DIO0"}, "Channel12"={"function"=enum."OFF", "switch high"=0.0, "switch low"=0.0, "scan begin"=0.0, "scan end"=0.0, "scan step"=0.0, "and gate high"=0.0, "and gate low"=0.0, "or gate high"=0.0, "or gate low"=0.0, "main input"=enum."DIO0", "sub input"=enum."DIO0"}, "Channel13"={"function"=enum."OFF", "switch high"=0.0, "switch low"=0.0, "scan begin"=0.0, "scan end"=0.0, "scan step"=0.0, "and gate high"=0.0, "and gate low"=0.0, "or gate high"=0.0, "or gate low"=0.0, "main input"=enum."DIO0", "sub input"=enum."DIO0"}, "Channel14"={"function"=enum."OFF", "switch high"=0.0, "switch low"=0.0, "scan begin"=0.0, "scan end"=0.0, "scan step"=0.0, "and gate high"=0.0, "and gate low"=0.0, "or gate high"=0.0, "or gate low"=0.0, "main input"=enum."DIO0", "sub input"=enum."DIO0"}, "Channel15"={"function"=enum."OFF", "switch high"=0.0, "switch low"=0.0, "scan begin"=0.0, "scan end"=0.0, "scan step"=0.0, "and gate high"=0.0, "and gate low"=0.0, "or gate high"=0.0, "or gate low"=0.0, "main input"=enum."DIO0", "sub input"=enum."DIO0"}} ("Output Configuration") -> [w13]
    shift-right: [w16] -> _
    shift-left: enum16{"Loading", "Running"}."Loading" ("State") -> [w15]
    shift-right: [w12] -> _
    shift-left: _ -> [w7]
    tunnel: w4 -> [w11]
    tunnel: w3 -> [w10]
    tunnel: [w9] -> w2
    tunnel: [w8] -> w1
    stop <- FALSE stop-if-true
    n3 = case shown="\"Running\"" w15 {
      selector: w15 -> [w92 w244]
      tunnel: [w91 w246] -> w16
      tunnel: [w85 w242] -> w14
      tunnel: w13 -> [w87 w242]
      tunnel: [w20 T1 {FALSE, FALSE, FALSE, FALSE, FALSE, FALSE, FALSE, FALSE, FALSE, FALSE, FALSE, FALSE, FALSE, FALSE, FALSE, FALSE}] -> w12
      tunnel: w11 -> [w19 w240]
      tunnel: w10 -> [w18 w239]
      tunnel: [w19 w238] -> w9
      tunnel: [w18 w237] -> w8
      tunnel: w7 -> [_ w232]
      frame "Loading", Default {
        n4 = Select(t=enum16{"Loading", "Running"}."Running", s="Load", f=w92) -> (s? t:f=w91:enum16{"Loading", "Running"})
        n5 = Select(t="Output Configuration", s="Load", f=w87) -> (s? t:f=w85:T2)
        n6 = Not Equal?(x="Output Configuration", y=w87) -> (x != y?=w89:T3)
        n7 = Unbundle(w89) -> ("Channel0"=w52:T4, "Channel1"=w51:T4, "Channel2"=w50:T4, "Channel3"=w49:T4, "Channel4"=w48:T4, "Channel5"=w47:T4, "Channel6"=w46:T4, "Channel7"=w45:T4, "Channel8"=w44:T4, "Channel9"=w43:T4, "Channel10"=w42:T4, "Channel11"=w41:T4, "Channel12"=w40:T4, "Channel13"=w39:T4, "Channel14"=w38:T4, "Channel15"=w37:T4)
        n8 = Cluster To Array(cluster=w52) -> (array=w62:bool[])
        n9 = Cluster To Array(cluster=w51) -> (array=w64:bool[])
        n10 = Cluster To Array(cluster=w50) -> (array=w66:bool[])
        n11 = Cluster To Array(cluster=w49) -> (array=w68:bool[])
        n12 = Cluster To Array(cluster=w48) -> (array=w70:bool[])
        n13 = Cluster To Array(cluster=w47) -> (array=w84:bool[])
        n14 = Cluster To Array(cluster=w46) -> (array=w80:bool[])
        n15 = Cluster To Array(cluster=w45) -> (array=w82:bool[])
        n16 = Cluster To Array(cluster=w44) -> (array=w78:bool[])
        n17 = Cluster To Array(cluster=w43) -> (array=w76:bool[])
        n18 = Cluster To Array(cluster=w42) -> (array=w74:bool[])
        n19 = Cluster To Array(cluster=w41) -> (array=w72:bool[])
        n20 = Cluster To Array(cluster=w40) -> (array=w60:bool[])
        n21 = Cluster To Array(cluster=w39) -> (array=w58:bool[])
        n22 = Cluster To Array(cluster=w38) -> (array=w56:bool[])
        n23 = Cluster To Array(cluster=w37) -> (array=w54:bool[])
        n24 = Boolean Array To Number(Boolean array=w62) -> (number=w61:u32)
        n25 = Boolean Array To Number(Boolean array=w64) -> (number=w63:u32)
        n26 = Boolean Array To Number(Boolean array=w66) -> (number=w65:u32)
        n27 = Boolean Array To Number(Boolean array=w68) -> (number=w67:u32)
        n28 = Boolean Array To Number(Boolean array=w70) -> (number=w69:u32)
        n29 = Boolean Array To Number(Boolean array=w84) -> (number=w83:u32)
        n30 = Boolean Array To Number(Boolean array=w80) -> (number=w79:u32)
        n31 = Boolean Array To Number(Boolean array=w82) -> (number=w81:u32)
        n32 = Boolean Array To Number(Boolean array=w78) -> (number=w77:u32)
        n33 = Boolean Array To Number(Boolean array=w76) -> (number=w75:u32)
        n34 = Boolean Array To Number(Boolean array=w74) -> (number=w73:u32)
        n35 = Boolean Array To Number(Boolean array=w72) -> (number=w71:u32)
        n36 = Boolean Array To Number(Boolean array=w60) -> (number=w59:u32)
        n37 = Boolean Array To Number(Boolean array=w58) -> (number=w57:u32)
        n38 = Boolean Array To Number(Boolean array=w56) -> (number=w55:u32)
        n39 = Boolean Array To Number(Boolean array=w54) -> (number=w53:u32)
        n40 = Not Equal To 0?(x=w61) -> (x != 0?=w36:bool)
        n41 = Not Equal To 0?(x=w63) -> (x != 0?=w35:bool)
        n42 = Not Equal To 0?(x=w65) -> (x != 0?=w34:bool)
        n43 = Not Equal To 0?(x=w67) -> (x != 0?=w33:bool)
        n44 = Not Equal To 0?(x=w69) -> (x != 0?=w32:bool)
        n45 = Not Equal To 0?(x=w83) -> (x != 0?=w31:bool)
        n46 = Not Equal To 0?(x=w79) -> (x != 0?=w30:bool)
        n47 = Not Equal To 0?(x=w81) -> (x != 0?=w29:bool)
        n48 = Not Equal To 0?(x=w77) -> (x != 0?=w28:bool)
        n49 = Not Equal To 0?(x=w75) -> (x != 0?=w27:bool)
        n50 = Not Equal To 0?(x=w73) -> (x != 0?=w26:bool)
        n51 = Not Equal To 0?(x=w71) -> (x != 0?=w25:bool)
        n52 = Not Equal To 0?(x=w59) -> (x != 0?=w24:bool)
        n53 = Not Equal To 0?(x=w57) -> (x != 0?=w23:bool)
        n54 = Not Equal To 0?(x=w55) -> (x != 0?=w22:bool)
        n55 = Not Equal To 0?(x=w53) -> (x != 0?=w21:bool)
        n56 = Bundle(w36, w35, w34, w33, w32, w31, w30, w29, w28, w27, w26, w25, w24, w23, w22, w21) -> (w20:T1)  [unwired: 1 in]
      }
      frame "Running" {
        n57 = Unbundle(w242) -> ("Channel0"=w241:T5, "Channel1"=w221:T5, "Channel2"=w212:T5, "Channel3"=w203:T5, "Channel4"=w175:T5, "Channel5"=w174:T5, "Channel6"=w173:T5, "Channel7"=w176:T5, "Channel8"=w139:T5, "Channel9"=w138:T5, "Channel10"=w137:T5, "Channel11"=w140:T5, "Channel12"=w103:T5, "Channel13"=w102:T5, "Channel14"=w101:T5, "Channel15"=w104:T5)
        n58 = Unbundle By Name(w241) -> ("function"=w236:T6, "main input"=w230:T7, "sub input"=w229:T7)
        n59 = Unbundle By Name(w221) -> ("function"=w227:T6, "main input"=w223:T7, "sub input"=w222:T7)
        n60 = Unbundle By Name(w212) -> ("function"=w218:T6, "main input"=w214:T7, "sub input"=w213:T7)
        n61 = Unbundle By Name(w203) -> ("function"=w209:T6, "main input"=w205:T7, "sub input"=w204:T7)
        n62 = Unbundle By Name(w175) -> ("function"=w200:T6, "main input"=w196:T7, "sub input"=w195:T7)
        n63 = Unbundle By Name(w174) -> ("function"=w194:T6, "main input"=w190:T7, "sub input"=w189:T7)
        n64 = Unbundle By Name(w173) -> ("function"=w188:T6, "main input"=w184:T7, "sub input"=w183:T7)
        n65 = Unbundle By Name(w176) -> ("function"=w182:T6, "main input"=w178:T7, "sub input"=w177:T7)
        n66 = Unbundle By Name(w139) -> ("function"=w164:T6, "main input"=w160:T7, "sub input"=w159:T7)
        n67 = Unbundle By Name(w138) -> ("function"=w158:T6, "main input"=w154:T7, "sub input"=w153:T7)
        n68 = Unbundle By Name(w137) -> ("function"=w152:T6, "main input"=w148:T7, "sub input"=w147:T7)
        n69 = Unbundle By Name(w140) -> ("function"=w146:T6, "main input"=w142:T7, "sub input"=w141:T7)
        n70 = Unbundle By Name(w103) -> ("function"=w128:T6, "main input"=w124:T7, "sub input"=w123:T7)
        n71 = Unbundle By Name(w102) -> ("function"=w122:T6, "main input"=w118:T7, "sub input"=w117:T7)
        n72 = Unbundle By Name(w101) -> ("function"=w116:T6, "main input"=w112:T7, "sub input"=w111:T7)
        n73 = Unbundle By Name(w104) -> ("function"=w110:T6, "main input"=w106:T7, "sub input"=w105:T7)
        n74 = case shown="\"ITERATION\"" w236 {
          tunnel: w241 -> [_ w539 w543 w547 w551]
          tunnel: [sgl 0.0 ("scan end") w538 w542 w546 w550] -> w235
          tunnel: [sgl 0.0 ("scan begin") w537 w541 w545 w549] -> w234
          tunnel: [sgl 0.0 ("scan step") sgl 0.0 ("scan step") sgl 0.0 ("scan step") sgl 0.0 ("scan step") w548] -> w233
          frame "OFF", Default {
          }
          frame "SWITCH" {
            n75 = Unbundle By Name(w539) -> ("switch high"=w538:sgl, "switch low"=w537:sgl)
          }
          frame "AND GATE" {
            n76 = Unbundle By Name(w543) -> ("and gate high"=w542:sgl, "and gate low"=w541:sgl)
          }
          frame "OR GATE" {
            n77 = Unbundle By Name(w547) -> ("or gate high"=w546:sgl, "or gate low"=w545:sgl)
          }
          frame "ITERATION" {
            n78 = Unbundle By Name(w551) -> ("scan begin"=w549:sgl, "scan end"=w550:sgl, "scan step"=w548:sgl)
          }
        }
        n79 = case shown="\"ITERATION\"" w227 {
          tunnel: w221 -> [_ w520 w524 w528 w532]
          tunnel: [sgl 0.0 ("scan end") w519 w523 w527 w531] -> w226
          tunnel: [sgl 0.0 ("scan begin") w518 w522 w526 w530] -> w225
          tunnel: [sgl 0.0 ("scan step") sgl 0.0 ("scan step") sgl 0.0 ("scan step") sgl 0.0 ("scan step") w529] -> w224
          frame "OFF", Default {
          }
          frame "SWITCH" {
            n80 = Unbundle By Name(w520) -> ("switch high"=w519:sgl, "switch low"=w518:sgl)
          }
          frame "AND GATE" {
            n81 = Unbundle By Name(w524) -> ("and gate high"=w523:sgl, "and gate low"=w522:sgl)
          }
          frame "OR GATE" {
            n82 = Unbundle By Name(w528) -> ("or gate high"=w527:sgl, "or gate low"=w526:sgl)
          }
          frame "ITERATION" {
            n83 = Unbundle By Name(w532) -> ("scan begin"=w530:sgl, "scan end"=w531:sgl, "scan step"=w529:sgl)
          }
        }
        n84 = case shown="\"ITERATION\"" w218 {
          tunnel: w212 -> [_ w501 w505 w509 w513]
          tunnel: [sgl 0.0 ("scan end") w500 w504 w508 w512] -> w217
          tunnel: [sgl 0.0 ("scan begin") w499 w503 w507 w511] -> w216
          tunnel: [sgl 0.0 ("scan step") sgl 0.0 ("scan step") sgl 0.0 ("scan step") sgl 0.0 ("scan step") w510] -> w215
          frame "OFF", Default {
          }
          frame "SWITCH" {
            n85 = Unbundle By Name(w501) -> ("switch high"=w500:sgl, "switch low"=w499:sgl)
          }
          frame "AND GATE" {
            n86 = Unbundle By Name(w505) -> ("and gate high"=w504:sgl, "and gate low"=w503:sgl)
          }
          frame "OR GATE" {
            n87 = Unbundle By Name(w509) -> ("or gate high"=w508:sgl, "or gate low"=w507:sgl)
          }
          frame "ITERATION" {
            n88 = Unbundle By Name(w513) -> ("scan begin"=w511:sgl, "scan end"=w512:sgl, "scan step"=w510:sgl)
          }
        }
        n89 = case shown="\"ITERATION\"" w209 {
          tunnel: w203 -> [_ w482 w486 w490 w494]
          tunnel: [sgl 0.0 ("scan end") w481 w485 w489 w493] -> w208
          tunnel: [sgl 0.0 ("scan begin") w480 w484 w488 w492] -> w207
          tunnel: [sgl 0.0 ("scan step") sgl 0.0 ("scan step") sgl 0.0 ("scan step") sgl 0.0 ("scan step") w491] -> w206
          frame "OFF", Default {
          }
          frame "SWITCH" {
            n90 = Unbundle By Name(w482) -> ("switch high"=w481:sgl, "switch low"=w480:sgl)
          }
          frame "AND GATE" {
            n91 = Unbundle By Name(w486) -> ("and gate high"=w485:sgl, "and gate low"=w484:sgl)
          }
          frame "OR GATE" {
            n92 = Unbundle By Name(w490) -> ("or gate high"=w489:sgl, "or gate low"=w488:sgl)
          }
          frame "ITERATION" {
            n93 = Unbundle By Name(w494) -> ("scan begin"=w492:sgl, "scan end"=w493:sgl, "scan step"=w491:sgl)
          }
        }
        n94 = case shown="\"ITERATION\"" w200 {
          tunnel: w175 -> [_ w463 w467 w471 w475]
          tunnel: [sgl 0.0 ("scan end") w462 w466 w470 w474] -> w199
          tunnel: [sgl 0.0 ("scan begin") w461 w465 w469 w473] -> w198
          tunnel: [sgl 0.0 ("scan step") sgl 0.0 ("scan step") sgl 0.0 ("scan step") sgl 0.0 ("scan step") w472] -> w197
          frame "OFF", Default {
          }
          frame "SWITCH" {
            n95 = Unbundle By Name(w463) -> ("switch high"=w462:sgl, "switch low"=w461:sgl)
          }
          frame "AND GATE" {
            n96 = Unbundle By Name(w467) -> ("and gate high"=w466:sgl, "and gate low"=w465:sgl)
          }
          frame "OR GATE" {
            n97 = Unbundle By Name(w471) -> ("or gate high"=w470:sgl, "or gate low"=w469:sgl)
          }
          frame "ITERATION" {
            n98 = Unbundle By Name(w475) -> ("scan begin"=w473:sgl, "scan end"=w474:sgl, "scan step"=w472:sgl)
          }
        }
        n99 = case shown="\"ITERATION\"" w194 {
          tunnel: w174 -> [_ w444 w448 w452 w456]
          tunnel: [sgl 0.0 ("scan end") w443 w447 w451 w455] -> w193
          tunnel: [sgl 0.0 ("scan begin") w442 w446 w450 w454] -> w192
          tunnel: [sgl 0.0 ("scan step") sgl 0.0 ("scan step") sgl 0.0 ("scan step") sgl 0.0 ("scan step") w453] -> w191
          frame "OFF", Default {
          }
          frame "SWITCH" {
            n100 = Unbundle By Name(w444) -> ("switch high"=w443:sgl, "switch low"=w442:sgl)
          }
          frame "AND GATE" {
            n101 = Unbundle By Name(w448) -> ("and gate high"=w447:sgl, "and gate low"=w446:sgl)
          }
          frame "OR GATE" {
            n102 = Unbundle By Name(w452) -> ("or gate high"=w451:sgl, "or gate low"=w450:sgl)
          }
          frame "ITERATION" {
            n103 = Unbundle By Name(w456) -> ("scan begin"=w454:sgl, "scan end"=w455:sgl, "scan step"=w453:sgl)
          }
        }
        n104 = case shown="\"ITERATION\"" w188 {
          tunnel: w173 -> [_ w425 w429 w433 w437]
          tunnel: [sgl 0.0 ("scan end") w424 w428 w432 w436] -> w187
          tunnel: [sgl 0.0 ("scan begin") w423 w427 w431 w435] -> w186
          tunnel: [sgl 0.0 ("scan step") sgl 0.0 ("scan step") sgl 0.0 ("scan step") sgl 0.0 ("scan step") w434] -> w185
          frame "OFF", Default {
          }
          frame "SWITCH" {
            n105 = Unbundle By Name(w425) -> ("switch high"=w424:sgl, "switch low"=w423:sgl)
          }
          frame "AND GATE" {
            n106 = Unbundle By Name(w429) -> ("and gate high"=w428:sgl, "and gate low"=w427:sgl)
          }
          frame "OR GATE" {
            n107 = Unbundle By Name(w433) -> ("or gate high"=w432:sgl, "or gate low"=w431:sgl)
          }
          frame "ITERATION" {
            n108 = Unbundle By Name(w437) -> ("scan begin"=w435:sgl, "scan end"=w436:sgl, "scan step"=w434:sgl)
          }
        }
        n109 = case shown="\"ITERATION\"" w182 {
          tunnel: w176 -> [_ w406 w410 w414 w418]
          tunnel: [sgl 0.0 ("scan end") w405 w409 w413 w417] -> w181
          tunnel: [sgl 0.0 ("scan begin") w404 w408 w412 w416] -> w180
          tunnel: [sgl 0.0 ("scan step") sgl 0.0 ("scan step") sgl 0.0 ("scan step") sgl 0.0 ("scan step") w415] -> w179
          frame "OFF", Default {
          }
          frame "SWITCH" {
            n110 = Unbundle By Name(w406) -> ("switch high"=w405:sgl, "switch low"=w404:sgl)
          }
          frame "AND GATE" {
            n111 = Unbundle By Name(w410) -> ("and gate high"=w409:sgl, "and gate low"=w408:sgl)
          }
          frame "OR GATE" {
            n112 = Unbundle By Name(w414) -> ("or gate high"=w413:sgl, "or gate low"=w412:sgl)
          }
          frame "ITERATION" {
            n113 = Unbundle By Name(w418) -> ("scan begin"=w416:sgl, "scan end"=w417:sgl, "scan step"=w415:sgl)
          }
        }
        n114 = case shown="\"ITERATION\"" w164 {
          tunnel: w139 -> [_ w387 w391 w395 w399]
          tunnel: [sgl 0.0 ("scan end") w386 w390 w394 w398] -> w163
          tunnel: [sgl 0.0 ("scan begin") w385 w389 w393 w397] -> w162
          tunnel: [sgl 0.0 ("scan step") sgl 0.0 ("scan step") sgl 0.0 ("scan step") sgl 0.0 ("scan step") w396] -> w161
          frame "OFF", Default {
          }
          frame "SWITCH" {
            n115 = Unbundle By Name(w387) -> ("switch high"=w386:sgl, "switch low"=w385:sgl)
          }
          frame "AND GATE" {
            n116 = Unbundle By Name(w391) -> ("and gate high"=w390:sgl, "and gate low"=w389:sgl)
          }
          frame "OR GATE" {
            n117 = Unbundle By Name(w395) -> ("or gate high"=w394:sgl, "or gate low"=w393:sgl)
          }
          frame "ITERATION" {
            n118 = Unbundle By Name(w399) -> ("scan begin"=w397:sgl, "scan end"=w398:sgl, "scan step"=w396:sgl)
          }
        }
        n119 = case shown="\"ITERATION\"" w158 {
          tunnel: w138 -> [_ w368 w372 w376 w380]
          tunnel: [sgl 0.0 ("scan end") w367 w371 w375 w379] -> w157
          tunnel: [sgl 0.0 ("scan begin") w366 w370 w374 w378] -> w156
          tunnel: [sgl 0.0 ("scan step") sgl 0.0 ("scan step") sgl 0.0 ("scan step") sgl 0.0 ("scan step") w377] -> w155
          frame "OFF", Default {
          }
          frame "SWITCH" {
            n120 = Unbundle By Name(w368) -> ("switch high"=w367:sgl, "switch low"=w366:sgl)
          }
          frame "AND GATE" {
            n121 = Unbundle By Name(w372) -> ("and gate high"=w371:sgl, "and gate low"=w370:sgl)
          }
          frame "OR GATE" {
            n122 = Unbundle By Name(w376) -> ("or gate high"=w375:sgl, "or gate low"=w374:sgl)
          }
          frame "ITERATION" {
            n123 = Unbundle By Name(w380) -> ("scan begin"=w378:sgl, "scan end"=w379:sgl, "scan step"=w377:sgl)
          }
        }
        n124 = case shown="\"ITERATION\"" w152 {
          tunnel: w137 -> [_ w349 w353 w357 w361]
          tunnel: [sgl 0.0 ("scan end") w348 w352 w356 w360] -> w151
          tunnel: [sgl 0.0 ("scan begin") w347 w351 w355 w359] -> w150
          tunnel: [sgl 0.0 ("scan step") sgl 0.0 ("scan step") sgl 0.0 ("scan step") sgl 0.0 ("scan step") w358] -> w149
          frame "OFF", Default {
          }
          frame "SWITCH" {
            n125 = Unbundle By Name(w349) -> ("switch high"=w348:sgl, "switch low"=w347:sgl)
          }
          frame "AND GATE" {
            n126 = Unbundle By Name(w353) -> ("and gate high"=w352:sgl, "and gate low"=w351:sgl)
          }
          frame "OR GATE" {
            n127 = Unbundle By Name(w357) -> ("or gate high"=w356:sgl, "or gate low"=w355:sgl)
          }
          frame "ITERATION" {
            n128 = Unbundle By Name(w361) -> ("scan begin"=w359:sgl, "scan end"=w360:sgl, "scan step"=w358:sgl)
          }
        }
        n129 = case shown="\"ITERATION\"" w146 {
          tunnel: w140 -> [_ w330 w334 w338 w342]
          tunnel: [sgl 0.0 ("scan end") w329 w333 w337 w341] -> w145
          tunnel: [sgl 0.0 ("scan begin") w328 w332 w336 w340] -> w144
          tunnel: [sgl 0.0 ("scan step") sgl 0.0 ("scan step") sgl 0.0 ("scan step") sgl 0.0 ("scan step") w339] -> w143
          frame "OFF", Default {
          }
          frame "SWITCH" {
            n130 = Unbundle By Name(w330) -> ("switch high"=w329:sgl, "switch low"=w328:sgl)
          }
          frame "AND GATE" {
            n131 = Unbundle By Name(w334) -> ("and gate high"=w333:sgl, "and gate low"=w332:sgl)
          }
          frame "OR GATE" {
            n132 = Unbundle By Name(w338) -> ("or gate high"=w337:sgl, "or gate low"=w336:sgl)
          }
          frame "ITERATION" {
            n133 = Unbundle By Name(w342) -> ("scan begin"=w340:sgl, "scan end"=w341:sgl, "scan step"=w339:sgl)
          }
        }
        n134 = case shown="\"ITERATION\"" w128 {
          tunnel: w103 -> [_ w311 w315 w319 w323]
          tunnel: [sgl 0.0 ("scan end") w310 w314 w318 w322] -> w127
          tunnel: [sgl 0.0 ("scan begin") w309 w313 w317 w321] -> w126
          tunnel: [sgl 0.0 ("scan step") sgl 0.0 ("scan step") sgl 0.0 ("scan step") sgl 0.0 ("scan step") w320] -> w125
          frame "OFF", Default {
          }
          frame "SWITCH" {
            n135 = Unbundle By Name(w311) -> ("switch high"=w310:sgl, "switch low"=w309:sgl)
          }
          frame "AND GATE" {
            n136 = Unbundle By Name(w315) -> ("and gate high"=w314:sgl, "and gate low"=w313:sgl)
          }
          frame "OR GATE" {
            n137 = Unbundle By Name(w319) -> ("or gate high"=w318:sgl, "or gate low"=w317:sgl)
          }
          frame "ITERATION" {
            n138 = Unbundle By Name(w323) -> ("scan begin"=w321:sgl, "scan end"=w322:sgl, "scan step"=w320:sgl)
          }
        }
        n139 = case shown="\"ITERATION\"" w122 {
          tunnel: w102 -> [_ w292 w296 w300 w304]
          tunnel: [sgl 0.0 ("scan end") w291 w295 w299 w303] -> w121
          tunnel: [sgl 0.0 ("scan begin") w290 w294 w298 w302] -> w120
          tunnel: [sgl 0.0 ("scan step") sgl 0.0 ("scan step") sgl 0.0 ("scan step") sgl 0.0 ("scan step") w301] -> w119
          frame "OFF", Default {
          }
          frame "SWITCH" {
            n140 = Unbundle By Name(w292) -> ("switch high"=w291:sgl, "switch low"=w290:sgl)
          }
          frame "AND GATE" {
            n141 = Unbundle By Name(w296) -> ("and gate high"=w295:sgl, "and gate low"=w294:sgl)
          }
          frame "OR GATE" {
            n142 = Unbundle By Name(w300) -> ("or gate high"=w299:sgl, "or gate low"=w298:sgl)
          }
          frame "ITERATION" {
            n143 = Unbundle By Name(w304) -> ("scan begin"=w302:sgl, "scan end"=w303:sgl, "scan step"=w301:sgl)
          }
        }
        n144 = case shown="\"ITERATION\"" w116 {
          tunnel: w101 -> [_ w273 w277 w281 w285]
          tunnel: [sgl 0.0 ("scan end") w272 w276 w280 w284] -> w115
          tunnel: [sgl 0.0 ("scan begin") w271 w275 w279 w283] -> w114
          tunnel: [sgl 0.0 ("scan step") sgl 0.0 ("scan step") sgl 0.0 ("scan step") sgl 0.0 ("scan step") w282] -> w113
          frame "OFF", Default {
          }
          frame "SWITCH" {
            n145 = Unbundle By Name(w273) -> ("switch high"=w272:sgl, "switch low"=w271:sgl)
          }
          frame "AND GATE" {
            n146 = Unbundle By Name(w277) -> ("and gate high"=w276:sgl, "and gate low"=w275:sgl)
          }
          frame "OR GATE" {
            n147 = Unbundle By Name(w281) -> ("or gate high"=w280:sgl, "or gate low"=w279:sgl)
          }
          frame "ITERATION" {
            n148 = Unbundle By Name(w285) -> ("scan begin"=w283:sgl, "scan end"=w284:sgl, "scan step"=w282:sgl)
          }
        }
        n149 = case shown="\"ITERATION\"" w110 {
          tunnel: w104 -> [_ w254 w258 w262 w266]
          tunnel: [sgl 0.0 ("scan end") w253 w257 w261 w265] -> w109
          tunnel: [sgl 0.0 ("scan begin") w252 w256 w260 w264] -> w108
          tunnel: [sgl 0.0 ("scan step") sgl 0.0 ("scan step") sgl 0.0 ("scan step") sgl 0.0 ("scan step") w263] -> w107
          frame "OFF", Default {
          }
          frame "SWITCH" {
            n150 = Unbundle By Name(w254) -> ("switch high"=w253:sgl, "switch low"=w252:sgl)
          }
          frame "AND GATE" {
            n151 = Unbundle By Name(w258) -> ("and gate high"=w257:sgl, "and gate low"=w256:sgl)
          }
          frame "OR GATE" {
            n152 = Unbundle By Name(w262) -> ("or gate high"=w261:sgl, "or gate low"=w260:sgl)
          }
          frame "ITERATION" {
            n153 = Unbundle By Name(w266) -> ("scan begin"=w264:sgl, "scan end"=w265:sgl, "scan step"=w263:sgl)
          }
        }
        n154 = Select(t=enum16{"Loading", "Running"}."Loading", s="Configure", f=w244) -> (s? t:f=w246:enum16{"Loading", "Running"})
        n155 = Unbundle(w232) -> (w231:bool, w219:bool, w211:bool, w202:bool, w172:bool, w171:bool, w170:bool, w169:bool, w136:bool, w135:bool, w134:bool, w133:bool, w100:bool, w99:bool, w98:bool, w97:bool)
        n156 = Bundle("function"=w236, "scan end"=w235, "scan begin"=w234, "scan step"=w233, w231, "main input"=w230, "sub input"=w229) -> (w228:T8)  [unwired: 1 in]
        n157 = Bundle("function"=w227, "scan end"=w226, "scan begin"=w225, "scan step"=w224, w219, "main input"=w223, "sub input"=w222) -> (w220:T8)  [unwired: 1 in]
        n158 = Bundle("function"=w218, "scan end"=w217, "scan begin"=w216, "scan step"=w215, w211, "main input"=w214, "sub input"=w213) -> (w210:T8)  [unwired: 1 in]
        n159 = Bundle("function"=w209, "scan end"=w208, "scan begin"=w207, "scan step"=w206, w202, "main input"=w205, "sub input"=w204) -> (w201:T8)  [unwired: 1 in]
        n160 = Bundle("function"=w200, "scan end"=w199, "scan begin"=w198, "scan step"=w197, w172, "main input"=w196, "sub input"=w195) -> (w168:T8)  [unwired: 1 in]
        n161 = Bundle("function"=w194, "scan end"=w193, "scan begin"=w192, "scan step"=w191, w171, "main input"=w190, "sub input"=w189) -> (w167:T8)  [unwired: 1 in]
        n162 = Bundle("function"=w188, "scan end"=w187, "scan begin"=w186, "scan step"=w185, w170, "main input"=w184, "sub input"=w183) -> (w166:T8)  [unwired: 1 in]
        n163 = Bundle("function"=w182, "scan end"=w181, "scan begin"=w180, "scan step"=w179, w169, "main input"=w178, "sub input"=w177) -> (w165:T8)  [unwired: 1 in]
        n164 = Bundle("function"=w164, "scan end"=w163, "scan begin"=w162, "scan step"=w161, w136, "main input"=w160, "sub input"=w159) -> (w132:T8)  [unwired: 1 in]
        n165 = Bundle("function"=w158, "scan end"=w157, "scan begin"=w156, "scan step"=w155, w135, "main input"=w154, "sub input"=w153) -> (w131:T8)  [unwired: 1 in]
        n166 = Bundle("function"=w152, "scan end"=w151, "scan begin"=w150, "scan step"=w149, w134, "main input"=w148, "sub input"=w147) -> (w130:T8)  [unwired: 1 in]
        n167 = Bundle("function"=w146, "scan end"=w145, "scan begin"=w144, "scan step"=w143, w133, "main input"=w142, "sub input"=w141) -> (w129:T8)  [unwired: 1 in]
        n168 = Bundle("function"=w128, "scan end"=w127, "scan begin"=w126, "scan step"=w125, w100, "main input"=w124, "sub input"=w123) -> (w96:T8)  [unwired: 1 in]
        n169 = Bundle("function"=w122, "scan end"=w121, "scan begin"=w120, "scan step"=w119, w99, "main input"=w118, "sub input"=w117) -> (w95:T8)  [unwired: 1 in]
        n170 = Bundle("function"=w116, "scan end"=w115, "scan begin"=w114, "scan step"=w113, w98, "main input"=w112, "sub input"=w111) -> (w94:T8)  [unwired: 1 in]
        n171 = Bundle("function"=w110, "scan end"=w109, "scan begin"=w108, "scan step"=w107, w97, "main input"=w106, "sub input"=w105) -> (w93:T8)  [unwired: 1 in]
        n172 = xnode "Read/Write Control"("FPGA VI Reference In"=w240, "error in"=w239, "Channel0"=w228, "Channel1"=w220, "Channel2"=w210, "Channel3"=w201, "Channel4"=w168, "Channel5"=w167, "Channel6"=w166, "Channel7"=w165, "Channel8"=w132, "Channel9"=w131, "Channel10"=w130, "Channel11"=w129, "Channel12"=w96, "Channel13"=w95, "Channel14"=w94, "Channel15"=w93) -> ("FPGA VI Reference Out"=w238:refnum<k20>, "error out"=w237:errorcluster)
      }
    }
    "change indicator" <- w12
    "State" <- w15
  }
  n173 = xnode "Close FPGA VI Reference"("FPGA VI Reference In"=w2, "error in"=w1) -> ()  [unwired: 1 out]
